vi "STED Control V7.vi"() -> ()   [LabVIEW 2014]
uses:
  Type Defs/Image Acquisition Parameters.ctl
  Laser Controls.ctl
  Detectors.ctl
  Type Defs/P541.ctl
  Type Defs/M227.ctl
  Type Defs/P612.ctl
  Type Defs/M686.ctl
  Type Defs/P841.ctl
  Type Defs/ASI.ctl
  Type Defs/N664_V2.ctl
  Type Defs/STED Graph Controls.ctl
  Type Defs/Display Controls.ctl
  FPGA-7842R-Reference.ctl
  Manual Controls V2.ctl
  Scan Parameters.ctl
  <vilib>/Utility/miscctls.llb/LVPositionTypeDef.ctl
  Controls/StageStates.ctl
  <vilib>/Utility/miscctls.llb/LVRectTypeDef.ctl
  <vilib>/Utility/cursorutil.llb/Set Cursor (Icon Pict).vi
panel:
  in  "Test":bool
  in  "Display Controls":T1
  in  "Graph Tools":T2
  in  "Shutters":T3
  in  "Upper Objective Z - N664":T4={"Up N664"=FALSE, "Down N664"=FALSE, "Step Size (um)"=0.001, "Position (mm)"=0.0} {"Step Size (um)" min=0.001}
  in  "Load Positions":bool
  in  "Cavity Translation Z - ASI":T5={"Up ASI"=FALSE, "Down ASI"=FALSE, "Step Size (um)"=0.001, "Z (um)"=0.001, "F (um)"=0.001, "Velocity"=0.001} caption="ASI" {"Velocity" min=0.001; "F (um)" min=0.001; "Z (um)" min=-1500.0 max=1500.0; "Step Size (um)" min=0.001}
  in  "Phase Comp Mirror - P841":T6={"Position (µm)"=0.0, "Step Size (µm)"=1.0, "Up P841"=FALSE, "Down P841"=FALSE}
  in  "Sample Stage XY - M686":T7 {"Y" format="%#_4g"; "X" format="%#_4g"}
  in  "Joystick Velocity":string(combo)
  in  "Radio Buttons":enum32{"Radio Selection 1", "Radio Selection 2"}(radio)
  in  "Bottom Objective XY - P612":T8 {"Y" format="%#_4g"; "X" format="%#_4g"}
  in  "Abort AllStage":bool
  in  "Stages":T9={"M227"=TRUE, "N664"=TRUE, "P612"=TRUE, "M686"=TRUE, "P841"=TRUE, "ASI"=TRUE}
  in  "Sample Z Coarse - M227":T10
  in  "Colormap":T11(ring)
  in  "Tab Control":T12(tab)
  in  "SLM":bool
  in  "DM":bool
  in  "Timing":bool
  in  "Sample Z - P541":T13={"Step Up"=FALSE, "Step Down"=FALSE, "Z Position"=0.0, "Step Size (um)"=1.0}
  out "Channel 6":sgl[][](graph)
  out "Channel 5":sgl[][](graph)
  out "Channel 4":sgl[][](graph)
  out "Channel 3":sgl[][](graph)
  out "Channel 2":sgl[][](graph)
  in  "Detectors":T14
  in  "Laser Controls":T15 {"STED Power (V)" scale=0.0..10.0}
  in  "Save File Path":path=path "C:/Users/ED STED/Desktop/temp.DBL"
  in  "Capture":bool
  out "Channel 1":sgl[][](graph)
  in  "Image Acquisition Parameters":T16={"Scan Type"=enum."Beam Scanning", "Scan Mode"=enum."XY", "Fast Axis Frequency (Hz)"=15780.0, "Image Format"=256, "Line Accumulations"=100, "Frames Per Capture"=1, "Frames Accumulations"=1, "Image Dimension (um)"=[15.0, 15.0], "Number of Z Steps"=1, "Z Steps Size (um)"=1.0, "Pixel Size (nm)"=[58.59375, 58.59375]} {"Z Steps Size (um)" min=0.0; "Number of Z Steps" min=1; "Frames Accumulations" min=1; "Frames Per Capture" min=1; "Line Accumulations" min=1; "Image Format" items=["64 x 64"=64, "128 x 128"=128, "256 x 256"=256, "512 x 512"=512, "1024 x 1024"=1024, "2048 x 2048"=2048]}
  in  "Live":bool
  in  "Exit":bool
  # "Sample Stage XY - M686 (0~25 mm)"
  # "XY"
  # "Z"
  # "Length"
  # "Height"
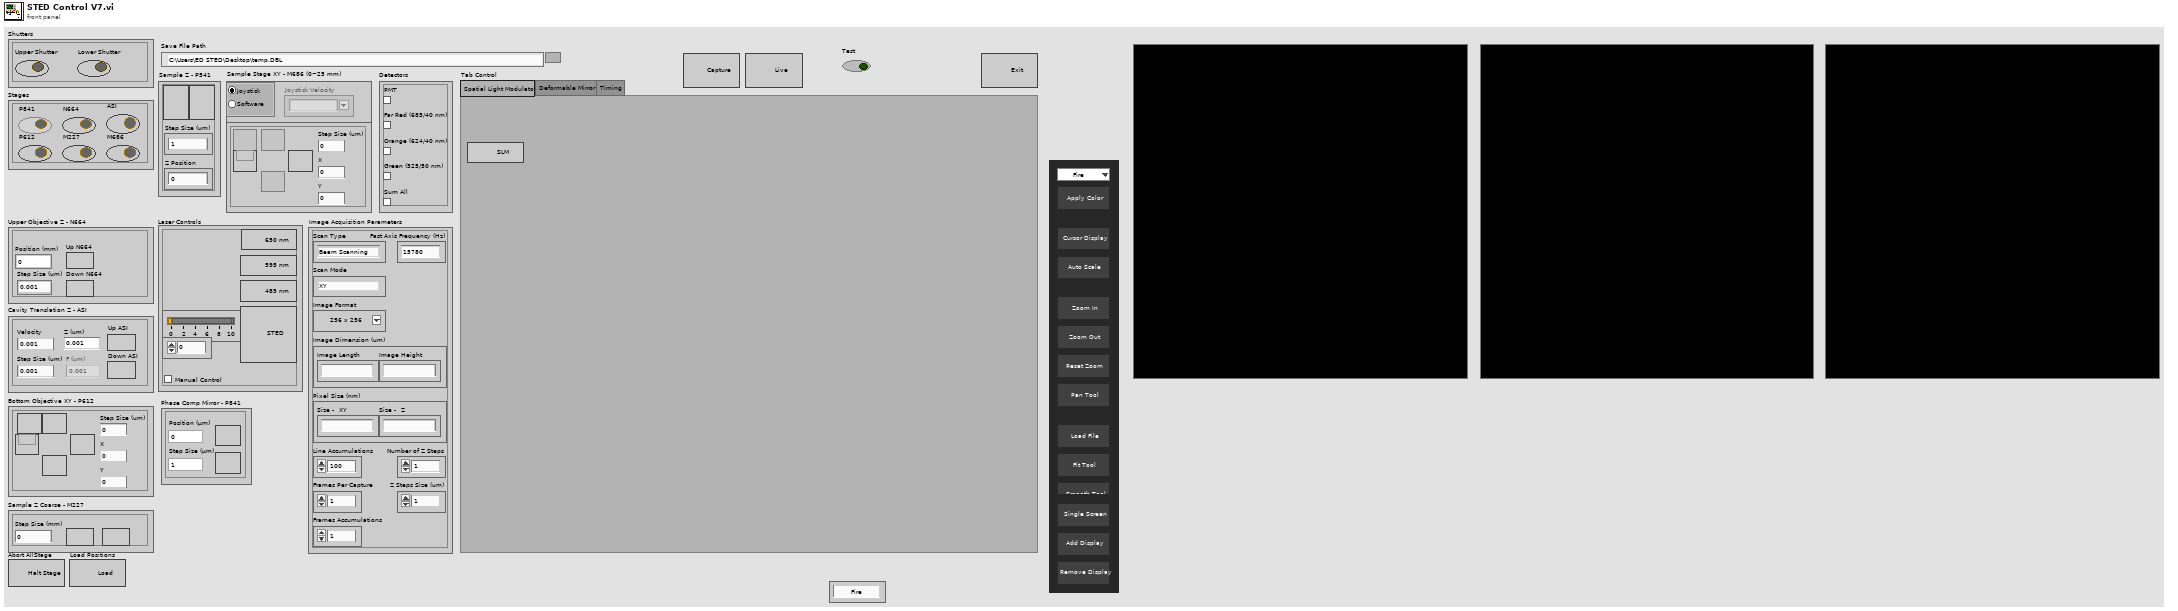
[diagram p1: front panel]
types:
  T1 = typedef "Display Controls.ctl" = cluster{"Remove Display":bool, "Add Display":bool, "Single Screen":bool}
  T2 = typedef "STED Graph Controls.ctl" = cluster{"Zoom Out":bool, "Zoom In":bool, "Reset Zoom":bool, "Pan Tool":bool, "Show Cursor":bool, "Load File":bool, "Fit Tool":bool, "Smooth Tool":bool, "Merge Tool":bool, "Auto Scale":bool, "Apply Color":bool, "Color Map":enum16{"Fire", "Gray", "Red", "Green", "Blue", "Cyan", "Magenta", "Yellow", "Red-White", "Green-White", "Blue-White", "Glow"}}
  T3 = cluster{"Upper Shutter":bool, "Lower Shutter":bool}
  T4 = typedef "N664_V2.ctl" = cluster{"Up N664":bool, "Down N664":bool, "Step Size (um)":dbl, "Position (mm)":dbl}
  T5 = typedef "ASI.ctl" = cluster{"Up ASI":bool, "Down ASI":bool, "Step Size (um)":dbl, "Z (um)":dbl, "F (um)":dbl, "Velocity":dbl}
  T6 = typedef "P841.ctl" = cluster{"Position (µm)":dbl, "Step Size (µm)":dbl, "Up P841":bool, "Down P841":bool}
  T7 = typedef "M686.ctl" = cluster{"Home Button":bool, "Up Button":bool, "Left Button":bool, "Down Button":bool, "Right Button":bool, "Step Size (um)":dbl, "X":dbl, "Y":dbl}
  T8 = typedef "P612.ctl" = cluster{"Home Button":bool, "Up Button":bool, "Left Button":bool, "Down Button":bool, "Right Button":bool, "Step Size (um)":dbl, "X":dbl, "Y":dbl}
  T9 = cluster{"M227":bool, "N664":bool, "P612":bool, "M686":bool, "P841":bool, "ASI":bool}
  T10 = typedef "M227.ctl" = cluster{"Up M227":bool, "Down M227":bool, "Step Size (mm)":dbl}
  T11 = enum16{"Fire", "Gray", "Red", "Green", "Blue", "Cyan", "Magenta", "Yellow", "Red-White", "Green-White", "Blue-White", "Glow"}
  T12 = enum32{"Spatial Light Modulator", "Deformable Mirror", "Timing"}
  T13 = typedef "P541.ctl" = cluster{"Step Up":bool, "Step Down":bool, "Z Position":dbl, "Step Size (um)":dbl}
  T14 = typedef "Detectors.ctl" = cluster{"PMT":bool, "Far Red (685/40 nm)":bool, "Orange (624/40 nm)":bool, "Green (525/50 nm)":bool, "Sum All":bool}
  T15 = typedef "Laser Controls.ctl" = cluster{"STED Power (V)":dbl, "STED":bool, "640 nm":bool, "590 nm":bool, "485 nm":bool, "Manual Control":bool}
  T16 = typedef "Image Acquisition Parameters.ctl" = cluster{"Scan Type":enum16{"Sample Scanning", "Beam Scanning"}, "Scan Mode":enum16{"XY", "XZ", "YZ", "XYZ"}, "Fast Axis Frequency (Hz)":dbl, "Image Format":u16, "Line Accumulations":u16, "Frames Per Capture":u16, "Frames Accumulations":u16, "Image Dimension (um)":dbl[], "Number of Z Steps":u8, "Z Steps Size (um)":dbl, "Pixel Size (nm)":dbl[]}
  T17 = typedef "Scan Parameters.ctl" = cluster{"Fast_Ax_Amp_V":dbl, "Fast_Ax_Off_V":dbl, "Slow_Ax_Amp_V":dbl, "Slow_Ax_Off_V ":dbl, "Slow_Ax_Max_V_VperS":dbl, "Slow_Ax1_Del25ns":i32, "Slow_Ax2_Del25ns":i32, "Stage_X_Off_V":dbl, "Stage_Y_Off_V":dbl, "Stage_Z_Off_V":dbl, "Galvo1_Off_V":dbl, "Galvo2_Off_V":dbl, "Last_Scan_Mode":enum16{"XY", "XZ", "YZ", "XYZ"}, "Current_Scan_Mode":enum16{"XY", "XZ", "YZ", "XYZ"}, "Fly_Back_Lines":u16, "Linear_Ramp_End":u32, "Z_Step_I16":i16, "Z_Start_I16":i16, "Laser_States _U32":u32, "590_Voltage_I16":i16, "775_AOM_Volt_I16":i16, "Blanking OFF":bool, "Unused_Axis_I16":i16}
  T18 = typedef "Manual Controls V2.ctl" = cluster{"Galvo 1 Position (I16)":i16, "Galvo 2 Position (I16)":i16, "X Axis Voltage (I16)":i16, "Y Axis Voltage (I16)":i16, "Z Axis Voltage (I16)":i16, "Res Mirror Amp (I16)":i16, "Res Mirror Mute":bool, "Upper Shutter":bool, "Lower Shutter":bool}
  T19 = typedef "FPGA-7842R-Reference.ctl" = enum16{"Stage Control", "Laser Control", "Unused Axis I16", "Exit", "Set Res Mirror", "Set Galvo", "Default", "Close FPGA", "Stop Waveforms", "Start Waveforms", "Shutter Control", "Initialize"}
  T20 = enum8{"Enabled", "Disabled", "Disabled and Grayed Out"}
  T21 = typedef "StageStates.ctl" = enum16{"POSITION", "MVR", "MOVE", "HALT", "ONTARGET", "ERROR", "EXIT", "HOME", "ZEROPOS", "NANOPOS", "QUIT", "ANALOG"}
  T22 = typedef "LVRectTypeDef.ctl" = cluster{"Left":i16, "Top":i16, "Right":i16, "Bottom":i16}
  T23 = enum32{"Invalid", "Standard", "Closed", "Hidden", "Minimized", "Maximized"}
  T24 = enum16{"open", "open or create", "create or replace", "create", "open (read-only)"}
  T25 = cluster{"Upper Shutter":bool, "Upper Shutter":bool}
  T26 = cluster{"Down_N664":bool, "Down_N664":bool, "Step Size (um)":dbl, "Numeric":dbl}
  T27 = cluster{bool, bool, bool, bool, bool, dbl, "Numeric":dbl, "Numeric":dbl}
  T28 = cluster{"Scan Type":bool, "Scan Mode":bool, "Fast Axis Frequency (Hz)":bool, "Image Format":bool, "Line Accumulations":bool, "Frames Per Capture":bool, "Frames Accumulations":bool, "Image Dimension (um)":bool[], "Number of Z Steps":bool, "Z Steps Size (um)":bool, "Pixel Size (nm)":bool[]}
  T29 = typedef "LVAllMonitorsDisplayTypeDef.ctl" = cluster{"Bounds":cluster{"Left":i16, "Top":i16, "Right":i16, "Bottom":i16}, "Depth":i16}[]
  T30 = cluster{"Bounds":cluster{"Left":i16, "Top":i16, "Right":i16, "Bottom":i16}, "Depth":i16}
  T31 = typedef "LVPositionTypeDef.ctl" = cluster{"Left":i32, "Top":i32}
  T32 = typedef "IMAQ Image.ctl" = refnum<image>
  T33 = typedef "Waveform Data.ctl" = cluster{"Waveform Scan Parameters":cluster{"Scanning Mode":u8, "Fast Axis WF Length (Elements)":i32, "Fast Axis Sample Period (Ticks)":u32, "Slow Axis 1 WF Length (Elements)":i32, "Slow Axis 1 Sample Period (Ticks)":u32, "Slow Axis 1 Delay (25 ns) Steps":i32, "Slow Axis 2 WFLength (Elements)":i32, "Slow Axis 2 Sample Period (Ticks)":u32, "Slow Axis 2 Delay (25 ns) Steps":i32}, "Fast Axis Waveform":dbl[], "Slow Axis 1 Waveform":dbl[], "Slow Axis 2 Waveform":dbl[]}
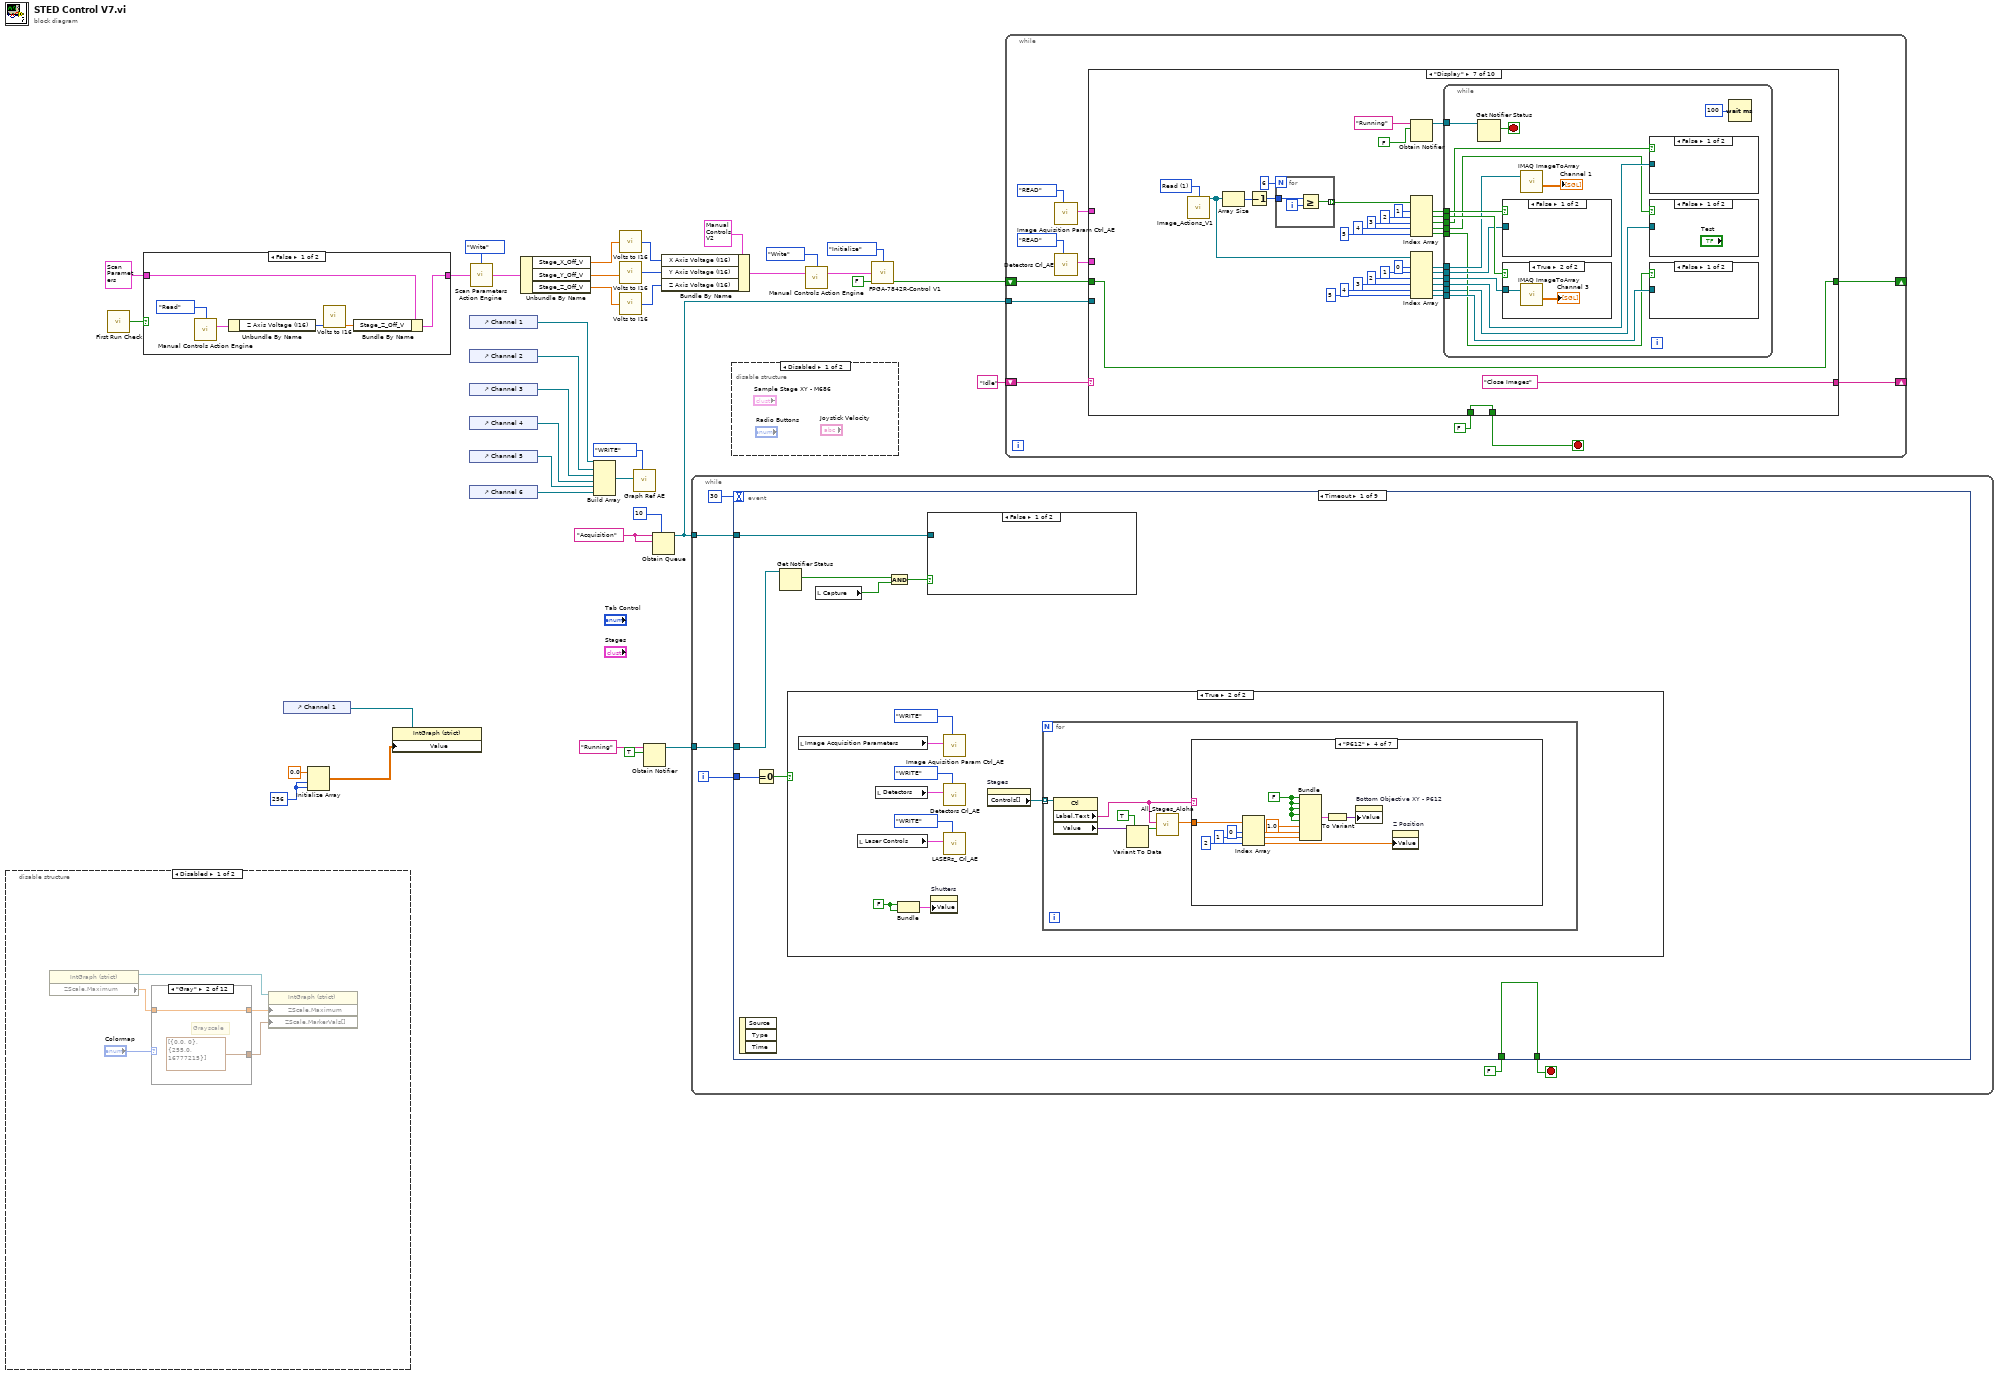
[diagram p0: block diagram]
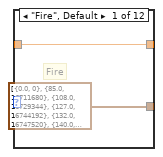
[diagram p2: hidden frame]
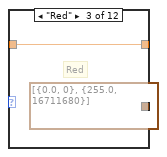
[diagram p3: hidden frame]
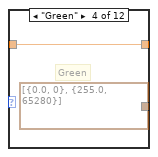
[diagram p4: hidden frame]
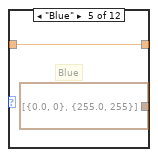
[diagram p5: hidden frame]
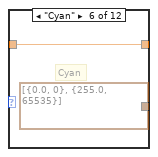
[diagram p6: hidden frame]
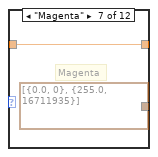
[diagram p7: hidden frame]
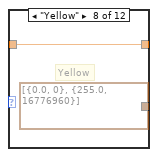
[diagram p8: hidden frame]
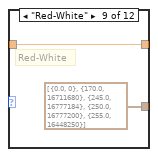
[diagram p9: hidden frame]
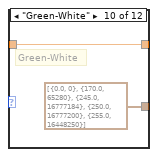
[diagram p10: hidden frame]
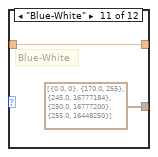
[diagram p11: hidden frame]
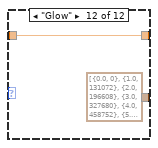
[diagram p12: hidden frame]
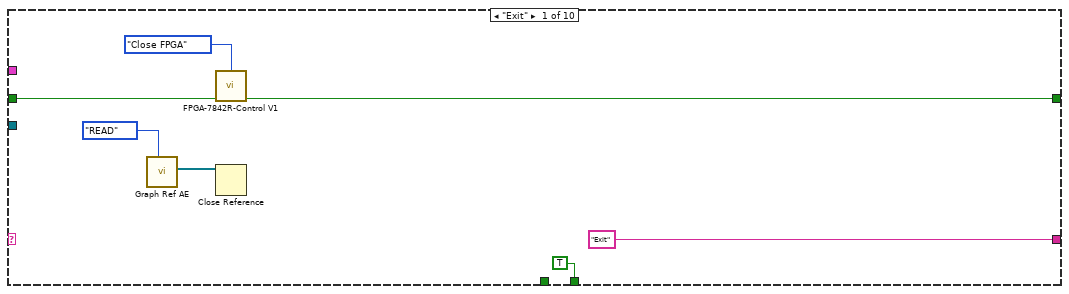
[diagram p16: hidden frame]
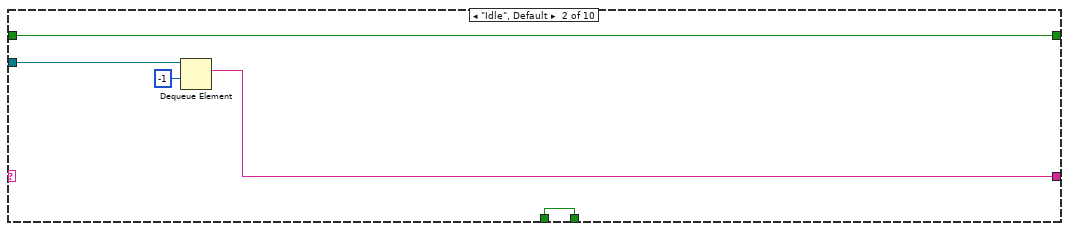
[diagram p17: hidden frame]
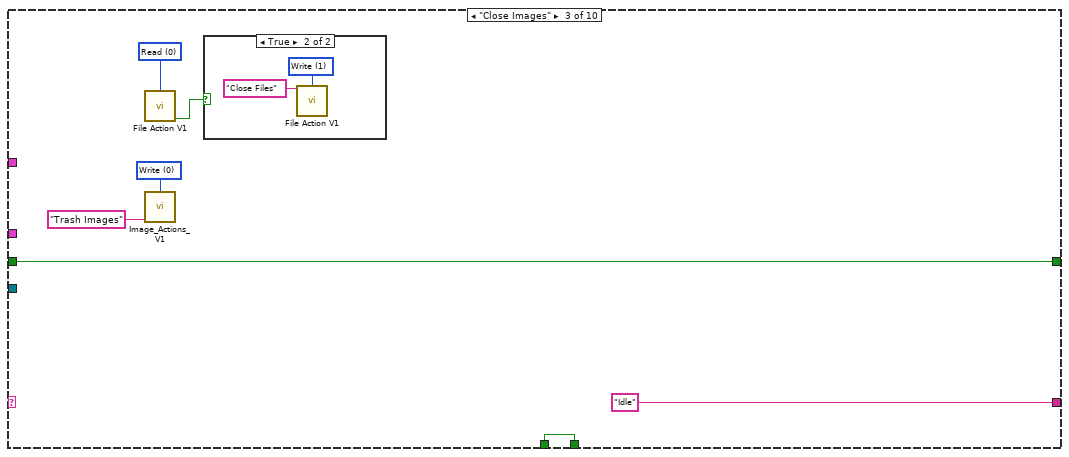
[diagram p18: hidden frame]
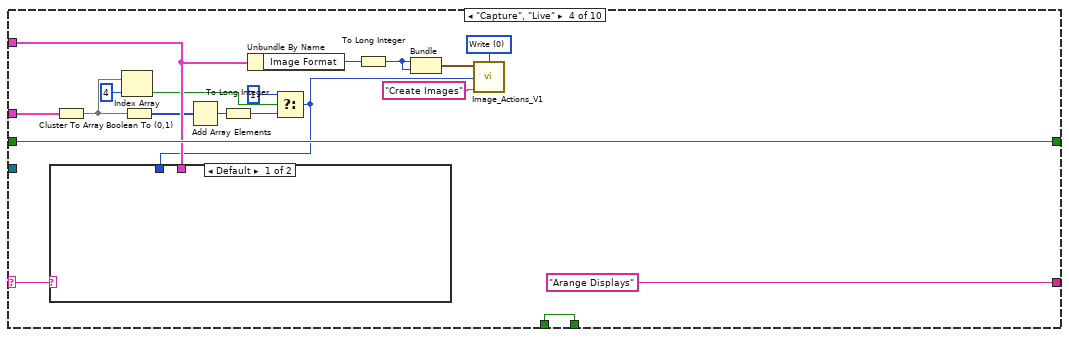
[diagram p20: hidden frame]
diagram:
  w3 = 256 ("dimension size")
  w14 = "Acquisition" ("name (unnamed)")
  n1 = disable-structure shown="Disabled" {
    frame Disabled {
      n2 = property class="IntGraph (strict)"() -> (reference out=w40:refnum<vi>, "ZScale.Maximum"=w39:dbl)  [unwired: 2 in, 1 out]
      n3 = case shown="\"Gray\"" "Colormap" {
        tunnel: [cluster{dbl, u32}[] [{0.0, 0}, {85.0, 16711680}, {108.0, 16729344}, {127.0, 16744192}, {132.0, 16747520}, {140.0, 16753920}, {157.0, 16766720}, {170.0, 16776960}, {245.0, 16777184}, {250.0, 16777200}, {255.0, 16777215}] ("Z Scale.Marker Values[]") cluster{dbl, u32}[] [{0.0, 0}, {255.0, 16777215}] ("Z Scale.Marker Values[]") cluster{dbl, u32}[] [{0.0, 0}, {255.0, 16711680}] ("Z Scale.Marker Values[]") cluster{dbl, u32}[] [{0.0, 0}, {255.0, 65280}] ("Z Scale.Marker Values[]") cluster{dbl, u32}[] [{0.0, 0}, {255.0, 255}] ("Z Scale.Marker Values[]") cluster{dbl, u32}[] [{0.0, 0}, {255.0, 65535}] ("Z Scale.Marker Values[]") cluster{dbl, u32}[] [{0.0, 0}, {255.0, 16711935}] ("Z Scale.Marker Values[]") cluster{dbl, u32}[] [{0.0, 0}, {255.0, 16776960}] ("Z Scale.Marker Values[]") cluster{dbl, u32}[] [{0.0, 0}, {170.0, 16711680}, {245.0, 16777184}, {250.0, 16777200}, {255.0, 16448250}] ("Z Scale.Marker Values[]") cluster{dbl, u32}[] [{0.0, 0}, {170.0, 65280}, {245.0, 16777184}, {250.0, 16777200}, {255.0, 16448250}] ("Z Scale.Marker Values[]") cluster{dbl, u32}[] [{0.0, 0}, {170.0, 255}, {245.0, 16777184}, {250.0, 16777200}, {255.0, 16448250}] ("Z Scale.Marker Values[]") cluster{dbl, u32}[] [{0.0, 0}, {1.0, 131072}, {2.0, 196608}, {3.0, 327680}, {4.0, 458752}, {5.0, 589824}, {6.0, 720896}, {7.0, 851971}, {8.0, 983043}, {9.0, 1114115}, {10.0, 1245187}, {11.0, 1376259}, {12.0, 1507331}, {13.0, 1638403}, {14.0, 1769475}, {15.0, 1769479}, {16.0, 2031623}, {17.0, 2162695}, {18.0, 2293767}, {19.0, 2424839}, {20.0, 2555911}, {21.0, 2686983}, {22.0, 2818055}, {23.0, 2949127}, {24.0, 3080203}, {25.0, 3211275}, {26.0, 3342347}, {27.0, 3473419}, {28.0, 3604491}, {29.0, 3735563}, {30.0, 3866635}, {31.0, 3867403}, {32.0, 4129547}, {33.0, 4260619}, {34.0, 4391691}, {35.0, 4522763}, {36.0, 4653839}, {37.0, 4784911}, {38.0, 4915983}, {39.0, 5178127}, {40.0, 5309199}, {41.0, 5440271}, {42.0, 5571343}, {43.0, 5702415}, {44.0, 5703439}, {45.0, 5965583}, {46.0, 6096655}, {47.0, 6227727}, {48.0, 6358799}, {49.0, 6489871}, {50.0, 6620943}, {51.0, 6752015}, {52.0, 6883087}, {53.0, 7015183}, {54.0, 7146255}, {55.0, 7277327}, {56.0, 7408399}, {57.0, 7539471}, {58.0, 7670543}, {59.0, 7801615}, {60.0, 8063759}, {61.0, 8194831}, {62.0, 8326927}, {63.0, 8457999}, {64.0, 8589075}, {65.0, 8720147}, {66.0, 8851219}, {67.0, 8982291}, {68.0, 9113363}, {69.0, 9114387}, {70.0, 9376531}, {71.0, 9507603}, {72.0, 9638675}, {73.0, 9769747}, {74.0, 9901843}, {75.0, 10032915}, {76.0, 10163987}, {77.0, 10229523}, {78.0, 10295059}, {79.0, 10427155}, {80.0, 10558227}, {81.0, 10689299}, {82.0, 10820371}, {83.0, 10886931}, {84.0, 10952467}, {85.0, 11083539}, {86.0, 11214611}, {87.0, 11215635}, {88.0, 11477779}, {89.0, 11543315}, {90.0, 11608851}, {91.0, 11740947}, {92.0, 11806483}, {93.0, 11872019}, {94.0, 12004115}, {95.0, 12135187}, {96.0, 12266259}, {97.0, 12267283}, {98.0, 12398355}, {99.0, 12529427}, {100.0, 12530451}, {101.0, 12595987}, {102.0, 12530451}, {103.0, 12793619}, {104.0, 12794131}, {105.0, 12794643}, {106.0, 13056787}, {107.0, 13057299}, {108.0, 13057811}, {109.0, 13188883}, {110.0, 13320979}, {111.0, 13386515}, {112.0, 13452563}, {113.0, 13584147}, {114.0, 13584659}, {115.0, 13585171}, {116.0, 13585683}, {117.0, 13717267}, {118.0, 13848339}, {119.0, 13849363}, {120.0, 13849875}, {121.0, 13850387}, {122.0, 13981459}, {123.0, 14113555}, {124.0, 14114067}, {125.0, 14114579}, {126.0, 14115091}, {127.0, 14246675}, {128.0, 14377747}, {129.0, 14378771}, {130.0, 14379283}, {131.0, 14379539}, {132.0, 14379795}, {133.0, 14380819}, {134.0, 14511891}, {135.0, 14643987}, {136.0, 14644503}, {137.0, 14645015}, {138.0, 14645527}, {139.0, 14646039}, {140.0, 14646551}, {141.0, 14778135}, {142.0, 14909207}, {143.0, 14910231}, {144.0, 14910747}, {145.0, 14911259}, {146.0, 14911771}, {147.0, 14912283}, {148.0, 14912797}, {149.0, 15044383}, {150.0, 15175455}, {151.0, 15175967}, {152.0, 15176479}, {153.0, 15176991}, {154.0, 15177507}, {155.0, 15178019}, {156.0, 15178531}, {157.0, 15310115}, {158.0, 15441701}, {159.0, 15441959}, {160.0, 15442215}, {161.0, 15442727}, {162.0, 15443243}, {163.0, 15443755}, {164.0, 15444269}, {165.0, 15444783}, {166.0, 15444783}, {167.0, 15576367}, {168.0, 15707953}, {169.0, 15708467}, {170.0, 15708979}, {171.0, 15708981}, {172.0, 15708983}, {173.0, 15710011}, {174.0, 15710523}, {175.0, 15711037}, {176.0, 15711039}, {177.0, 15711553}, {178.0, 15843139}, {179.0, 15974213}, {180.0, 15974215}, {181.0, 15974217}, {182.0, 15974219}, {183.0, 15975755}, {184.0, 15976271}, {185.0, 15976785}, {186.0, 15977299}, {187.0, 15977301}, {188.0, 15977815}, {189.0, 15978327}, {190.0, 15978331}, {191.0, 16109917}, {192.0, 16241503}, {193.0, 16241505}, {194.0, 16242019}, {195.0, 16242535}, {196.0, 16242537}, {197.0, 16242539}, {198.0, 16243563}, {199.0, 16243567}, {200.0, 16244081}, {201.0, 16244595}, {202.0, 16244599}, {203.0, 16244601}, {204.0, 16244603}, {205.0, 16245627}, {206.0, 16245631}, {207.0, 16245633}, {208.0, 16246147}, {209.0, 16246663}, {210.0, 16377735}, {211.0, 16508811}, {212.0, 16508815}, {213.0, 16509839}, {214.0, 16509843}, {215.0, 16509845}, {216.0, 16509847}, {217.0, 16510361}, {218.0, 16510875}, {219.0, 16510879}, {220.0, 16510881}, {221.0, 16510883}, {222.0, 16511399}, {223.0, 16511911}, {224.0, 16511915}, {225.0, 16511917}, {226.0, 16511919}, {227.0, 16511923}, {228.0, 16512437}, {229.0, 16512951}, {230.0, 16512955}, {231.0, 16512957}, {232.0, 16512959}, {233.0, 16512961}, {234.0, 16512963}, {235.0, 16512967}, {236.0, 16513481}, {237.0, 16513995}, {238.0, 16513999}, {239.0, 16514001}, {240.0, 16514003}, {241.0, 16514005}, {242.0, 16514007}, {243.0, 16514011}, {244.0, 16514013}, {245.0, 16514015}, {246.0, 16514019}, {247.0, 16514021}, {248.0, 16514023}, {249.0, 16514027}, {250.0, 16514029}, {251.0, 16514031}, {252.0, 16514035}, {253.0, 16514037}, {254.0, 16514039}, {255.0, 16514043}] ("Z Scale.Marker Values[]")] -> w42
        tunnel: [w43 w45 w47 w49 w51 w53 w55 w57 w59 w61 w63 w65] -> w41
        tunnel: w39 -> [w43 w45 w47 w49 w51 w53 w55 w57 w59 w61 w63 w65]
        frame "Fire", Default {
          # "Fire"
        }
        frame "Gray" {
          # "Grayscale"
        }
        frame "Red" {
          # "Red"
        }
        frame "Green" {
          # "Green"
        }
        frame "Blue" {
          # "Blue"
        }
        frame "Cyan" {
          # "Cyan"
        }
        frame "Magenta" {
          # "Magenta"
        }
        frame "Yellow" {
          # "Yellow"
        }
        frame "Red-White" {
          # "Red-White"
        }
        frame "Green-White" {
          # "Green-White"
        }
        frame "Blue-White" {
          # "Blue-White"
        }
        frame "Glow" {
        }
      }
      n4 = property class="IntGraph (strict)"(reference=w40, "ZScale.Maximum"=w41, "ZScale.MarkerVals[]"=w42) -> ()  [unwired: 1 in, 2 out]
    }
    frame Enabled {
    }
  }
  n5 = call "First Run Check.vi"() -> ("First Run?"=w7:bool)  [unwired: 15 in]
  n6 = case shown="False" w7 {
    tunnel: T17 {"Fast_Ax_Amp_V"=0.0, "Fast_Ax_Off_V"=0.0, "Slow_Ax_Amp_V"=0.0, "Slow_Ax_Off_V "=0.0, "Slow_Ax_Max_V_VperS"=0.0, "Slow_Ax1_Del25ns"=0, "Slow_Ax2_Del25ns"=0, "Stage_X_Off_V"=5.0, "Stage_Y_Off_V"=5.0, "Stage_Z_Off_V"=5.0, "Galvo1_Off_V"=0.0, "Galvo2_Off_V"=0.0, "Last_Scan_Mode"=enum."XY", "Current_Scan_Mode"=enum."XY", "Fly_Back_Lines"=0, "Linear_Ramp_End"=0, "Z_Step_I16"=0, "Z_Start_I16"=0, "Laser_States _U32"=0, "590_Voltage_I16"=0, "775_AOM_Volt_I16"=0, "Blanking OFF"=FALSE, "Unused_Axis_I16"=16384} ("Scan Parameters IN") -> [w72 w73]
    tunnel: [w67 w73] -> w5
    frame False {
      n7 = call "Manual Controls Action Engine.vi"("Action"=enum16{"Read", "Write"}."Read") -> ("Manual Controls Out"=w70:T18)  [unwired: 14 in]
      n8 = Unbundle By Name(w70) -> ("Z Axis Voltage (I16)"=w71:i16)
      n9 = call "Volts to I16.vi"("Volatge (I16)"=w71) -> ("Voltage (V)"=w68:dbl)  [unwired: 13 in, 1 out]
      n10 = Bundle By Name(cluster=w72, "Stage_Z_Off_V"=w68) -> (w67:T17)
    }
    frame True {
    }
  }
  n11 = control-ref of="Channel 1"() -> (w4:refnum<vi>)
  n12 = Initialize Array(sgl 0.0 ("element"), w3, w3) -> (w1:sgl[][])
  n13 = property class="IntGraph (strict)"(reference=w4, "Value"=w1) -> ()  [unwired: 1 in, 2 out]
  n14 = control-ref of="Channel 1"() -> (w8:refnum<vi>)
  n15 = control-ref of="Channel 2"() -> (w34:refnum<vi>)
  n16 = control-ref of="Channel 3"() -> (w19:refnum<vi>)
  n17 = control-ref of="Channel 4"() -> (w33:refnum<vi>)
  n18 = control-ref of="Channel 5"() -> (w32:refnum<vi>)
  n19 = control-ref of="Channel 6"() -> (w31:refnum<vi>)
  n20 = call "Scan Parameters Action Engine.vi"("Action"=enum16{"Read", "Write"}."Write", "Scan Parameters IN"=w5) -> ("Scan Parameters OUT"=w26:T17)  [unwired: 13 in]
  n21 = Unbundle By Name(w26) -> ("Stage_X_Off_V"=w22:dbl, "Stage_Y_Off_V"=w21:dbl, "Stage_Z_Off_V"=w20:dbl)
  n22 = Build Array(w8, w34, w19, w33, w32, w31) -> (w17:refnum<vi>[])
  n23 = call "Volts to I16.vi"("Voltage (V)"=w22) -> ("I16"=w23:i16)  [unwired: 13 in, 1 out]
  n24 = call "Volts to I16.vi"("Voltage (V)"=w21) -> ("I16"=w24:i16)  [unwired: 13 in, 1 out]
  n25 = call "Volts to I16.vi"("Voltage (V)"=w20) -> ("I16"=w25:i16)  [unwired: 13 in, 1 out]
  n26 = call "Graph Ref AE.vi"("Action"=enum16{"READ", "WRITE"}."WRITE", "Graph Ref In"=w17) -> ()  [unwired: 9 in, 1 out]
  n27 = Obtain Notifier(name (unnamed)="Running", notification data type=TRUE) -> (notifier out=w10:refnum<notifier>)  [unwired: 2 in, 2 out]
  n28 = Obtain Queue(max queue size (-1, unlimited)=10, name (unnamed)=w14, element data type=w14) -> (queue out=w16:refnum<queue>)  [unwired: 2 in, 2 out]
  n29 = Bundle By Name(cluster=T18 {"Galvo 1 Position (I16)"=-280, "Galvo 2 Position (I16)"=0, "X Axis Voltage (I16)"=16384, "Y Axis Voltage (I16)"=16384, "Z Axis Voltage (I16)"=16384, "Res Mirror Amp (I16)"=0, "Res Mirror Mute"=FALSE, "Upper Shutter"=FALSE, "Lower Shutter"=FALSE} ("Manual Controls"), "X Axis Voltage (I16)"=w23, "Y Axis Voltage (I16)"=w24, "Z Axis Voltage (I16)"=w25) -> (w27:T18)
  n30 = while {
    tunnel: w16 -> [w77]
    tunnel: w10 -> [w74]
    i -> [w75]
    stop <- w79 stop-if-true
    n31 = event shown="[0] Timeout" {
      selector: _ -> [_ _ _ _ _ _ _ _ _]
      dyn-events: _ -> [_ _ _ _ _ _ _ _ _]
      timeout: 30 -> [_ _ _ _ _ _ _ _ _]
      tunnel: [w87 w187 w200 w323 w552 w603 _ w784 w885] -> w79
      tunnel: FALSE -> [w87 w187 w200 w323 w552 w603 _ w784 _]
      tunnel: w77 -> [w84 w186 _ _ _ _ _ _ w884]
      tunnel: w75 -> [w82 _ _ _ _ _ _ _ _]
      tunnel: w74 -> [w80 w179 _ _ _ _ _ _ w878]
      event Timeout {
        n32 = event-data() -> ()  [unwired: 1 in, 3 out]
        n33 = Equal To 0?(x=w82) -> (x = 0?=w81:bool)
        n34 = Get Notifier Status(notifier=w80) -> (current notification=w86:bool)  [unwired: 1 in, 4 out]
        n35 = case shown="True" w81 {
          frame False {
            w92 = enum16{"WRITE", "READ"}."READ" ("Enum")
            n36 = call "Image Aquisition Param Ctrl_AE.vi"("Action"=enum16{"READ", "WRITE"}."READ") -> ("Image Acquisition Parameters Out"=w108:T16)  [unwired: 10 in]
            n37 = call "Detectors Crl_AE.vi"("Action"=enum16{"READ", "WRITE"}."READ") -> ("Detectors Parameters Out"=w109:T14)  [unwired: 10 in]
            n38 = call "LASERs_ Crl_AE.vi"("Action"=enum16{"READ", "WRITE"}."READ") -> ("Detectors Parameters Out"=w110:T15)  [unwired: 10 in]
            n39 = local write "Image Acquisition Parameters"(w108) -> ()
            n40 = local write "Detectors"(w109) -> ()
            n41 = local write "Laser Controls"(w110) -> ()
            n42 = call "Stage_position_ae.vi"("StageID"="P612", "Enum"=w92) -> ("Position Out"=w103:dbl[])  [unwired: 8 in, 1 out]
            n43 = call "Stage_position_ae.vi"("StageID"="P841", "Enum"=w92) -> ("Position Out"=w96:dbl[])  [unwired: 8 in, 1 out]
            n44 = call "Stage_position_ae.vi"("StageID"="N664", "Enum"=w92) -> ("Position Out"=w89:dbl[])  [unwired: 8 in, 1 out]
            n45 = Index Array(array=w89, index=0) -> (element=w88:dbl)
            n46 = Index Array(array=w96, index=0) -> (element=w93:dbl)
            n47 = Index Array(array=w103, index #1=0 ("index"), index #2=1 ("index"), index #3=2 ("index")) -> (element #1=w102:dbl, element #2=w99:dbl, element #3=w97:dbl)
            n48 = property on="Position (µm)" class="DigNum (strict)"("Value"=w93) -> ()  [unwired: 2 in, 2 out]
            n49 = property on="Position (mm)" class="DigNum (strict)"("Value"=w88) -> ()  [unwired: 2 in, 2 out]
            n50 = property on="X" class="DigNum (strict)"("Value"=w102) -> ()  [unwired: 2 in, 2 out]
            n51 = property on="Y" class="DigNum (strict)"("Value"=w99) -> ()  [unwired: 2 in, 2 out]
            n52 = property on="Z Position" class="DigNum (strict)"("Value"=w97) -> ()  [unwired: 2 in, 2 out]
          }
          frame True {
            w111 = FALSE ("Upper Shutter")
            n53 = local read "Image Acquisition Parameters"() -> (w118:T16)
            n54 = local read "Laser Controls"() -> (w116:T15)
            n55 = local read "Detectors"() -> (w115:T14)
            n56 = Bundle("Upper Shutter"=w111, "Upper Shutter"=w111) -> (w112:T25)  [unwired: 1 in]
            n57 = property on="Shutters" class="Clust (strict)"("Value"=w112) -> ()  [unwired: 2 in, 2 out]
            n58 = call "Image Aquisition Param Ctrl_AE.vi"("Action"=enum16{"READ", "WRITE"}."WRITE", "Image Acquisition Parameters In"=w118) -> ()  [unwired: 9 in, 1 out]
            n59 = call "Detectors Crl_AE.vi"("Action"=enum16{"READ", "WRITE"}."WRITE", "Detectors Parameters In"=w115) -> ()  [unwired: 9 in, 1 out]
            n60 = call "LASERs_ Crl_AE.vi"("Action"=enum16{"READ", "WRITE"}."WRITE", "Detectors Parameters In"=w116) -> ()  [unwired: 9 in, 1 out]
            n61 = property on="Stages" class="Clust (strict)"() -> ("Controls[]"=w113:refnum<vi>[])  [unwired: 2 in, 2 out]
            n62 = for {
              tunnel: w113 -> [w123] mode=indexing
              n63 = property class="Ctl"(reference=w123) -> ("Label.Text"=w121:string, "Value"=w125:variant)  [unwired: 1 in, 2 out]
              n64 = Variant To Data(type=TRUE, Variant=w125) -> (data=w122:bool)  [unwired: 1 in, 1 out]
              n65 = call "All_Stages_Aloha.vi"("Aloha"=w122, "Stage ID"=w121) -> ("Position Out"=w120:dbl[])  [unwired: 9 in]
              n66 = case shown="\"P612\"" w121 {
                tunnel: w120 -> [_ _ w132 w139 w149 w160 w170]
                frame "0", Default {
                }
                frame "M227" {
                  w129 = FALSE
                  n67 = Bundle(w129, w129, 0.0) -> (w127:cluster{bool, bool, dbl})  [unwired: 1 in]
                  n68 = To Variant(anything=w127) -> (Variant=w126:variant)
                  n69 = property on="Sample Z Coarse - M227" class="Clust"("Value"=w126) -> ()  [unwired: 2 in, 2 out]
                }
                frame "N664" {
                  w135 = FALSE ("Down_N664")
                  n70 = Index Array(array=w132, index=0) -> (element=w133:dbl)
                  n71 = Bundle("Down_N664"=w135, "Down_N664"=w135, "Step Size (um)"=1.0, "Numeric"=w133) -> (w131:T26)  [unwired: 1 in]
                  n72 = To Variant(anything=w131) -> (Variant=w130:variant)
                  n73 = property on="Upper Objective Z - N664" class="Clust"("Value"=w130) -> ()  [unwired: 2 in, 2 out]
                }
                frame "P612" {
                  w147 = FALSE
                  n74 = Index Array(array=w139, index #1=0, index #2=1, index #3=2 ("index")) -> (element #1=w144:dbl, element #2=w142:dbl, element #3=w137:dbl)
                  n75 = Bundle(w147, w147, w147, w147, w147, 1.0, "Numeric"=w144, "Numeric"=w142) -> (w143:T27)  [unwired: 1 in]
                  n76 = To Variant(anything=w143) -> (Variant=w138:variant)
                  n77 = property on="Bottom Objective XY - P612" class="Clust"("Value"=w138) -> ()  [unwired: 2 in, 2 out]
                  n78 = property on="Z Position" class="DigNum (strict)"("Value"=w137) -> ()  [unwired: 2 in, 2 out]
                }
                frame "M686" {
                  w158 = FALSE
                  n79 = Index Array(array=w149, index #1=0, index #2=1) -> (element #1=w155:dbl, element #2=w150:dbl)
                  n80 = Bundle(w158, w158, w158, w158, w158, 10.0, "Numeric"=w155, "Numeric"=w150) -> (w154:T27)  [unwired: 1 in]
                  n81 = To Variant(anything=w154) -> (Variant=w148:variant)
                  n82 = property on="Joystick Velocity" class="CmbBox"("DisabledEnum"=T20."Disabled and Grayed Out" ("Disabled")) -> ()  [unwired: 2 in, 2 out]
                  n83 = property on="Radio Buttons" class="RadioBtnsControl (strict)"("Value"=enum32{"Radio Selection 1", "Radio Selection 2"}."Radio Selection 2" ("Radio Buttons")) -> ()  [unwired: 2 in, 2 out]
                  n84 = property on="Sample Stage XY - M686" class="Clust"("Value"=w148) -> ()  [unwired: 2 in, 2 out]
                }
                frame "P841" {
                  n85 = Index Array(array=w160, index=0) -> (element=w159:dbl)
                  n86 = property on="Position (µm)" class="DigNum (strict)"("Value"=w159) -> ()  [unwired: 2 in, 2 out]
                }
                frame "ASI" {
                  w166 = FALSE
                  n87 = Add Array Elements(numeric array=w170) -> (sum=w172:dbl)
                  n88 = Index Array(array=w170, index #1=0 ("index"), index #2=1 ("index")) -> (element #1=w165:dbl, element #2=w164:dbl)
                  n89 = Divide(x=w172, y=2000.0) -> ()  [unwired: 1 out]
                  n90 = Bundle By Name(cluster=T5 {"Up ASI"=FALSE, "Down ASI"=FALSE, "Step Size (um)"=0.001, "Z (um)"=0.001, "F (um)"=0.001, "Velocity"=0.001} ("Cavity Translation Z - ASI"), "Up ASI"=w166, "Down ASI"=w166, "Step Size (um)"=1.0, "Z (um)"=w165, "F (um)"=w164, "Velocity"=0.1) -> (w162:T5)
                  n91 = To Variant(anything=w162) -> (Variant=w163:variant)
                  n92 = property on="Cavity Translation Z - ASI" class="Clust"("Value"=w163) -> ()  [unwired: 2 in, 2 out]
                }
              }
            }
          }
        }
        n93 = local read "Capture"() -> (w85:bool)
        n94 = And(x=w86, y=w85) -> (x .and. y?=w83:bool)
        n95 = case shown="False" w83 {
          tunnel: w84 -> [_ w177]
          frame False {
          }
          frame True {
            n96 = local write "Capture"(FALSE ("Capture")) -> ()
            n97 = Enqueue Element(queue=w177, element="Stop Acquisition" ("f")) -> ()  [unwired: 2 in, 3 out]
            n98 = property on="Live" class="Bool (strict)"("DisabledEnum"=T20."Enabled" ("Disabled")) -> ()  [unwired: 2 in, 2 out]
          }
        }
      }
      event "Live", "Capture": Value Change {
        n99 = event-data() -> ("CtlRef"=w185:refnum<vi>, "NewVal"=w180:bool)  [unwired: 1 in]
        n100 = Not(x=w180) -> (.not. x?=w183:bool)
        n101 = property class="Bool (strict)"(reference=w185) -> ("Label.Text"=w181:string)  [unwired: 1 in, 2 out]
        n102 = Send Notification(notification=w183, notifier=w179) -> ()  [unwired: 1 in, 2 out]
        n103 = case shown="\"Capture\"" w181 {
          tunnel: w180 -> [_ w189 w193]
          frame "False", Default {
          }
          frame "Live" {
            n104 = case shown="True" w189 {
              tunnel: [T20."Enabled" ("Disabled") T20."Disabled and Grayed Out" ("Disabled")] -> w188
              frame False {
              }
              frame True {
              }
            }
            n105 = property on="Capture" class="Bool (strict)"("DisabledEnum"=w188) -> ()  [unwired: 2 in, 2 out]
            n106 = property on="Exit" class="Bool"("DisabledEnum"=w188) -> ()  [unwired: 2 in, 2 out]
          }
          frame "Capture" {
            n107 = case shown="True" w193 {
              tunnel: [T20."Enabled" ("Disabled") T20."Disabled and Grayed Out" ("Disabled")] -> w192
              frame False {
              }
              frame True {
              }
            }
            n108 = property on="Live" class="Bool (strict)"("DisabledEnum"=w192) -> ()  [unwired: 2 in, 2 out]
            n109 = property on="Exit" class="Bool"("DisabledEnum"=w192) -> ()  [unwired: 2 in, 2 out]
          }
        }
        n110 = Select(t=w181, s=w180, f="Stop Acquisition") -> (s? t:f=w182:string)
        n111 = Enqueue Element(queue=w186, element=w182) -> ()  [unwired: 2 in, 3 out]
      }
      event "Shutters": Value Change {
        n112 = event-data() -> ("CtlRef"=w199:refnum<vi>, "NewVal"=w198:variant, "OldVal"=w197:variant)  [unwired: 1 in]
        n113 = property class="Clust"(reference=w199) -> ("Label.Text"=w196:string)  [unwired: 1 in, 2 out]
        n114 = case shown="\"Shutters\"" w196 {
          tunnel: w198 -> [_ w205 _ _ _]
          tunnel: w197 -> [_ w203 _ _ _]
          frame Default {
          }
          frame "Image Acquisition Parameters" {
            n115 = Variant To Data(type="Image Acquisition Parameters", Variant=w205) -> (data=w202:T16)  [unwired: 1 in, 1 out]
            n116 = Variant To Data(type=w202, Variant=w203) -> (data=w201:T16)  [unwired: 1 in, 1 out]
            n117 = Not Equal?(x=w202, y=w201) -> (x != y?=w227:T28)
            n118 = Unbundle By Name(w227) -> ("Image Dimension (um)"=w212:bool[], "Image Format"=w210:bool, "Pixel Size (nm)"=w211:bool[])
            n119 = Or Array Elements(Boolean array=w212) -> (logical OR=w216:bool)
            n120 = Or Array Elements(Boolean array=w211) -> (logical OR=w215:bool)
            n121 = Build Array(w216, w210, w215) -> (w214:bool[])
            n122 = Boolean Array To Number(Boolean array=w214) -> (number=w213:u32)
            n123 = case shown="0, Default" w213 {
              tunnel: w212 -> [_ w251 _]
              tunnel: w202 -> [w239 w244 w259]
              tunnel: [w239 w242 w257] -> w209
              tunnel: w211 -> [_ _ w256]
              tunnel: [w238 w241 w255] -> w208
              tunnel: [w237 w240 w254] -> w206
              frame 0, Default {
                n124 = Unbundle By Name(w239) -> ("Image Dimension (um)"=w238:dbl[], "Scan Mode"=w237:enum16{"XY", "XZ", "YZ", "XYZ"})
              }
              frame 1, 2 {
                # "Image Dimension or Format Change"
                n125 = Unbundle By Name(w244) -> ("Image Dimension (um)"=w250:dbl[], "Image Format"=w248:u16, "Scan Mode"=w240:enum16{"XY", "XZ", "YZ", "XYZ"})
                n126 = for {
                  tunnel: w251 -> [w253] mode=indexing
                  tunnel: w250 -> [w252] mode=indexing
                  tunnel: [w252] -> w249
                  stop <- w253 stop-if-true
                }
                n127 = To Double Precision Float(number=w248) -> (double precision float=w247:dbl)
                n128 = Build Array(w249, w249) -> (w241:dbl[])
                n129 = Divide(x=w241, y=w247) -> (x/y=w246:dbl[])
                n130 = Multiply(x=w246, y=1000.0) -> (x*y=w243:dbl[])
                n131 = Bundle By Name(cluster=w244, "Image Dimension (um)"=w241, "Pixel Size (nm)"=w243) -> (w242:T16)
              }
              frame 4 {
                # "Pixel Size Change"
                n132 = Unbundle By Name(w259) -> ("Pixel Size (nm)"=w265:dbl[], "Image Format"=w263:u16, "Scan Mode"=w254:enum16{"XY", "XZ", "YZ", "XYZ"})
                n133 = for {
                  tunnel: w256 -> [w267] mode=indexing
                  tunnel: w265 -> [w266] mode=indexing
                  tunnel: [w266] -> w264
                  stop <- w267 stop-if-true
                }
                n134 = Build Array(w264, w264) -> (w258:dbl[])
                n135 = To Double Precision Float(number=w263) -> (double precision float=w262:dbl)
                n136 = Multiply(x=w258, y=w262) -> (x*y=w261:dbl[])
                n137 = Multiply(x=w261, y=0.001) -> (x*y=w255:dbl[])
                n138 = Bundle By Name(cluster=w259, "Pixel Size (nm)"=w258, "Image Dimension (um)"=w255) -> (w257:T16)
              }
            }
            n139 = Index Array(array=w208, index=0) -> (element=w232:dbl)
            n140 = Not Equal?(x=enum16{"XY", "XZ", "YZ", "XYZ"}."YZ" ("y"), y=w206) -> (x != y?=w217:bool)
            n141 = call "Res Mirror um to Volts.vi"("Image Size (um)"=w232) -> ("Voltage (V)"=w233:dbl)
            n142 = Select(t=15780.0, s=w217, f=200.0) -> (s? t:f=w220:dbl)
            n143 = In Range and Coerce(upper limit=5.0, x=w233, lower limit=0.0) -> (coerced(x)=w234:dbl)  [unwired: 1 out]
            n144 = Bundle By Name(cluster=w209, "Fast Axis Frequency (Hz)"=w220) -> (w219:T16)
            n145 = call "Volts to I16.vi"("Voltage (V)"=w234) -> ("I16"=w231:i16)  [unwired: 13 in, 1 out]
            n146 = call "Manual Controls Action Engine.vi"("Action"=enum16{"Read", "Write"}."Read") -> ("Manual Controls Out"=w225:T18)  [unwired: 14 in]
            n147 = Bundle By Name(cluster=w225, "Res Mirror Amp (I16)"=w231, "Res Mirror Mute"=w217) -> (w223:T18)
            n148 = call "Image Aquisition Param Ctrl_AE.vi"("Action"=enum16{"READ", "WRITE"}."WRITE", "Image Acquisition Parameters In"=w219) -> ()  [unwired: 9 in, 1 out]
            n149 = call "FPGA-7842R-Control V1.vi"("Action"=FPGA-7842R-Reference."Set Res Mirror", "Manual Controls"=w223, "Initialize"=TRUE) -> ()  [unwired: 11 in, 2 out]
            n150 = call "Manual Controls Action Engine.vi"("Action"=enum16{"Read", "Write"}."Write", "Manual Controls In"=w223) -> ()  [unwired: 13 in, 1 out]
          }
          frame "Detectors" {
            n151 = call "Detectors Crl_AE.vi"("Action"=enum16{"READ", "WRITE"}."WRITE", "Detectors Parameters In"="Detectors") -> ()  [unwired: 9 in, 1 out]
          }
          frame "Laser Controls" {
            w282 = FALSE ("element")
            n152 = Unbundle By Name("Laser Controls") -> ("STED"=w288:bool, "640 nm"=w285:bool, "590 nm"=w286:bool, "485 nm"=w287:bool, "STED Power (V)"=w279:dbl, "Manual Control"=w273:bool)
            n153 = local read "Live"() -> (w274:bool)
            n154 = call "LASERs_ Crl_AE.vi"("Action"=enum16{"READ", "WRITE"}."WRITE", "Detectors Parameters In"="Laser Controls") -> ()  [unwired: 9 in, 1 out]
            n155 = Or(x=w274, y=w273) -> (x .or. y?=w272:bool)
            n156 = In Range and Coerce(upper limit=10.0, x=w279, lower limit=0.0) -> (coerced(x)=w276:dbl)  [unwired: 1 out]
            n157 = Build Array(w288, w285, w286, w287, w282, w282, w282, w282) -> (w284:bool[])
            n158 = case shown="True" w272 {
              tunnel: "Laser Controls" -> [_ w294]
              frame False {
              }
              frame True {
                n159 = call "FPGA-7842R-Control V1.vi"("Action"=FPGA-7842R-Reference."Laser Control", "Laser Controls"=w294, "Initialize"=TRUE) -> ()  [unwired: 11 in, 2 out]
              }
            }
            n160 = Boolean Array To Number(Boolean array=w284) -> (number=w283:u32)
            n161 = To Unsigned Byte Integer(number=w283) -> (unsigned 8bit integer=w281:u8)
            n162 = call "U8_To_U32.vi"("U8 IN"=w281) -> ("U32 OUT"=w280:u32)  [unwired: 13 in, 1 out]
            n163 = call "Volts to I16.vi"("Voltage (V)"=w276) -> ("I16"=w275:i16)  [unwired: 13 in, 1 out]
            n164 = call "Scan Parameters Action Engine.vi"("Action"=enum16{"Read", "Write"}."Read") -> ("Scan Parameters OUT"=w291:T17)  [unwired: 14 in]
            n165 = Bundle By Name(cluster=w291, "Laser_States _U32"=w280, "775_AOM_Volt_I16"=w275) -> (w289:T17)
            n166 = call "Scan Parameters Action Engine.vi"("Action"=enum16{"Read", "Write"}."Write", "Scan Parameters IN"=w289) -> ()  [unwired: 13 in, 1 out]
          }
          frame "Shutters" {
            n167 = Unbundle By Name("Shutters") -> ("Upper Shutter"=w306:bool, "Lower Shutter"=w305:bool)
            n168 = Not(x=w306) -> (.not. x?=w297:bool)
            n169 = Not(x=w305) -> (.not. x?=w296:bool)
            n170 = call "Manual Controls Action Engine.vi"("Action"=enum16{"Read", "Write"}."Read") -> ("Manual Controls Out"=w301:T18)  [unwired: 14 in]
            n171 = Bundle By Name(cluster=w301, "Upper Shutter"=w297, "Lower Shutter"=w296) -> (w298:T18)
            n172 = call "Manual Controls Action Engine.vi"("Action"=enum16{"Read", "Write"}."Write", "Manual Controls In"=w298) -> ()  [unwired: 13 in, 1 out]
            n173 = call "FPGA-7842R-Control V1.vi"("Action"=FPGA-7842R-Reference."Shutter Control", "Manual Controls"=w298, "Initialize"=TRUE) -> ()  [unwired: 11 in, 2 out]
          }
        }
      }
      event Value Change {
        # "For P541 - Sample Z - Converting from Step in µm to I16 is as follows. We have (Step µw)*(10 V / 100 µm)*(32768 I16 / 10 V) = (Step µm)*(32768 I16 / 100 µm) = (Step µm)*(327.68 I16/µm)"
        n174 = event-data() -> ("CtlRef"=w321:refnum<vi>, "OldVal"=w319:variant, "NewVal"=w320:variant)  [unwired: 1 in]
        n175 = local write "Abort AllStage"(FALSE ("Abort AllStage")) -> ()
        n176 = property class="Clust"(reference=w321) -> ("Label.Text"=w318:string, "ClassName"=w307:string)  [unwired: 1 in, 2 out]
        n177 = case shown="\"Upper Objective Z - N664\"" w318 {
          tunnel: w320 -> [_ w344 w372 w399 w462 w489 w515]
          tunnel: w319 -> [_ w343 w371 w398 w463 w490 w516]
          tunnel: ["" "N664" "ASI" "P612" "P612" "P841" "M227"] -> w317
          tunnel: [dbl[] [0.0] w335 w364 w387 dbl[] [0.0] w478 w505] -> w316
          tunnel: [bool[] [FALSE] w333 w358 w388 bool[] [FALSE] bool[] [TRUE] w507] -> w315
          tunnel: [enum16{"MOVE", "MVR"}."MVR" ("MOVE/MVR") w332 w361 w390 enum16{"MOVE", "MVR"}."MVR" ("MOVE/MVR") w481 enum16{"MOVE", "MVR"}."MVR" ("MOVE/MVR")] -> w314
          tunnel: [0.0 ("Step Size (um)") 0.5 ("Step Size (um)") w363 0.0 ("Velocity") 0.0 ("Velocity") 10000.0 ("Velocity") 0.0 ("Velocity")] -> w310
          tunnel: [StageStates."MVR" ("Action") w330 w362 w391 StageStates."POSITION" ("Action") w482 StageStates."MVR" ("Action")] -> w308
          frame Default {
          }
          frame "Upper Objective Z - N664" {
            n178 = call "N664_Ctrl_Index.vi"("OldVal"=w343, "NewVal"=w344) -> ("Control Ref OUT"=w342:refnum<vi>, "N664 Out"=w340:T4)  [unwired: 12 in]
            n179 = property class="Ctl"(reference=w342) -> ("Label.Text"=w341:string)  [unwired: 1 in, 2 out]
            n180 = Unbundle By Name(w340) -> ("Step Size (um)"=w339:dbl, "Position (mm)"=w338:dbl)
            n181 = case shown="\"Down N664\"" w341 {
              tunnel: w339 -> [_ w350 w354 _]
              tunnel: [0.0 ("Step Size (um)") w350 w353 w357] -> w336
              tunnel: w338 -> [_ _ _ w357]
              tunnel: [enum16{"MOVE", "MVR"}."MVR" ("MOVE/MVR") enum16{"MOVE", "MVR"}."MVR" ("MOVE/MVR") enum16{"MOVE", "MVR"}."MVR" ("MOVE/MVR") enum16{"MOVE", "MVR"}."MOVE" ("MOVE/MVR")] -> w332
              tunnel: [StageStates."MVR" ("Action") StageStates."MVR" ("Action") StageStates."MVR" ("Action") StageStates."MOVE" ("Action")] -> w330
              frame Default {
              }
              frame "Up N664" {
              }
              frame "Down N664" {
                n182 = Negate(x=w354) -> (-x=w353:dbl)
              }
              frame "Position (mm)" {
              }
            }
            n183 = Build Array(w336) -> (w335:dbl[])
            n184 = Build Array(TRUE) -> (w333:bool[])
          }
          frame "Cavity Translation Z - ASI" {
            n185 = call "ASI_Ctrl_Index.vi"("NewVal"=w372, "OldVal"=w371) -> ("ASI out"=w368:T5, "Control Ref OUT"=w370:refnum<vi>)  [unwired: 8 in]
            n186 = property class="Ctl"(reference=w370) -> ("Label.Text"=w369:string)  [unwired: 1 in, 2 out]
            n187 = Unbundle By Name(w368) -> ("Step Size (um)"=w367:dbl, "Z (um)"=w366:dbl, "Velocity"=w363:dbl)
            n188 = case shown="\"Down ASI\"" w369 {
              tunnel: w367 -> [_ w378 w381 _]
              tunnel: w366 -> [_ _ _ w385]
              tunnel: [0.0 ("Z (um)") w378 w382 w385] -> w365
              tunnel: [StageStates."MVR" ("Action") StageStates."MVR" ("Action") StageStates."MVR" ("Action") StageStates."MOVE" ("Action")] -> w362
              tunnel: [enum16{"MOVE", "MVR"}."MVR" ("MOVE/MVR") enum16{"MOVE", "MVR"}."MVR" ("MOVE/MVR") enum16{"MOVE", "MVR"}."MVR" ("MOVE/MVR") enum16{"MOVE", "MVR"}."MOVE" ("MOVE/MVR")] -> w361
              frame Default {
              }
              frame "Up ASI" {
              }
              frame "Down ASI" {
                n189 = Negate(x=w381) -> (-x=w382:dbl)
              }
              frame "Z (um)" {
              }
            }
            n190 = Build Array(w365) -> (w364:dbl[])
            n191 = Build Array(TRUE) -> (w358:bool[])
          }
          frame "Bottom Objective XY - P612" {
            n192 = call "P612_Ctrl_Index.vi"("OldVal"=w398, "NewVal"=w399) -> ("Control out"=w397:refnum<vi>, "P612 out"=w395:T8)  [unwired: 12 in]
            n193 = property class="Ctl"(reference=w397) -> ("Label.Text"=w396:string)  [unwired: 1 in, 2 out]
            n194 = Unbundle By Name(w395) -> ("Step Size (um)"=w394:dbl, "X"=w393:dbl, "Y"=w392:dbl)
            n195 = case shown="\"Up Button\"" w396 {
              tunnel: w394 -> [_ _ w410 w417 w421 w428 _]
              tunnel: w393 -> [_ _ _ _ _ _ w435]
              tunnel: w392 -> [_ _ _ _ _ _ w434]
              tunnel: [StageStates."MVR" ("Action") StageStates."HOME" ("Action") StageStates."MVR" ("Action") StageStates."MVR" ("Action") StageStates."MVR" ("Action") StageStates."MVR" ("Action") StageStates."MOVE" ("Action")] -> w391
              tunnel: [enum16{"MOVE", "MVR"}."MVR" ("MOVE/MVR") enum16{"MOVE", "MVR"}."MVR" ("MOVE/MVR") enum16{"MOVE", "MVR"}."MVR" ("MOVE/MVR") enum16{"MOVE", "MVR"}."MVR" ("MOVE/MVR") enum16{"MOVE", "MVR"}."MVR" ("MOVE/MVR") enum16{"MOVE", "MVR"}."MVR" ("MOVE/MVR") enum16{"MOVE", "MVR"}."MOVE" ("MOVE/MVR")] -> w390
              tunnel: [bool[] [FALSE] bool[] [TRUE, TRUE] bool[] [TRUE, FALSE] bool[] [TRUE, FALSE] bool[] [FALSE, TRUE] bool[] [FALSE, TRUE] bool[] [TRUE, TRUE]] -> w388
              tunnel: [dbl[] [0.0] dbl[] [0.0, 0.0] w409 w416 w423 w430 w436] -> w387
              frame Default {
              }
              frame "Home Button" {
              }
              frame "Up Button" {
                n196 = Build Array(w410, 0.0 ("element")) -> (w409:dbl[])
              }
              frame "Down Button" {
                n197 = Negate(x=w417) -> (-x=w414:dbl)
                n198 = Build Array(w414, 0.0 ("element")) -> (w416:dbl[])
              }
              frame "Left Button" {
                n199 = Build Array(0.0 ("element"), w421) -> (w423:dbl[])
              }
              frame "Right Button" {
                n200 = Negate(x=w428) -> (-x=w427:dbl)
                n201 = Build Array(0.0 ("element"), w427) -> (w430:dbl[])
              }
              frame "X", "Y" {
                n202 = Build Array(w435, w434) -> (w436:dbl[])
              }
            }
          }
          frame "Sample Z - P541" {
            w455 = 327.68 ("y")
            n203 = call "P541_Ctrl_Index.vi"("OldVal"=w463, "NewVal"=w462) -> ("Control out"=w461:refnum<vi>, "P541 Out"=w460:T13)  [unwired: 12 in]
            n204 = property class="Ctl"(reference=w461) -> ("Label.Text"=w458:string)  [unwired: 1 in, 2 out]
            n205 = Unbundle By Name(w460) -> ("Z Position"=w456:dbl, "Step Size (um)"=w459:dbl)
            n206 = call "Manual Controls Action Engine.vi"("Action"=enum16{"Read", "Write"}."Read") -> ("Manual Controls Out"=w447:T18)  [unwired: 14 in]
            n207 = Unbundle By Name(w447) -> ("Z Axis Voltage (I16)"=w450:i16)
            n208 = Multiply(x=w455, y=w456) -> (x*y=w453:dbl)
            n209 = Multiply(x=w459, y=w455) -> (x*y=w457:dbl)
            n210 = Round To Nearest(number=w453) -> (nearest integer value=w442:dbl)
            n211 = Round To Nearest(number=w457) -> (nearest integer value=w441:dbl)
            n212 = To Word Integer(number=w442) -> (16bit integer=w452:i16)
            n213 = To Word Integer(number=w441) -> (16bit integer=w454:i16)
            n214 = case shown="\"Step Down\"" w458 {
              tunnel: w454 -> [_ w470 w474 _]
              tunnel: w452 -> [_ _ _ w476]
              tunnel: w450 -> [w469 w472 w475 _]
              tunnel: [w469 w471 w473 w476] -> w446
              frame Default {
              }
              frame "Step Down" {
                n215 = Subtract(x=w472, y=w470) -> (x-y=w471:i16)
              }
              frame "Step Up" {
                n216 = Add(x=w475, y=w474) -> (x+y=w473:i16)
              }
              frame "Z Position" {
              }
            }
            n217 = Bundle By Name(cluster=w447, "Z Axis Voltage (I16)"=w446) -> (w449:T18)
            n218 = call "Manual Controls Action Engine.vi"("Action"=enum16{"Read", "Write"}."Write", "Manual Controls In"=w449) -> ("Manual Controls Out"=w443:T18)  [unwired: 13 in]
            n219 = call "FPGA-7842R-Control V1.vi"("Action"=FPGA-7842R-Reference."Stage Control", "Manual Controls"=w443, "Initialize"=TRUE) -> ()  [unwired: 11 in, 2 out]
          }
          frame "Phase Comp Mirror - P841" {
            n220 = call "P841_Ctrl_Index.vi"("OldVal"=w490, "NewVal"=w489) -> ("Control out"=w487:refnum<vi>, "P841 Out"=w485:T6)  [unwired: 12 in]
            n221 = property class="Ctl"(reference=w487) -> ("Label.Text"=w486:string)  [unwired: 1 in, 2 out]
            n222 = Unbundle By Name(w485) -> ("Position (µm)"=w484:dbl, "Step Size (µm)"=w483:dbl)
            n223 = case shown="\"Down P841\"" w486 {
              tunnel: w484 -> [_ _ _ w503]
              tunnel: w483 -> [_ w496 w500 _]
              tunnel: [0.0 ("Position (µm)") w496 w499 w503] -> w479
              tunnel: [StageStates."MVR" ("Action") StageStates."MVR" ("Action") StageStates."MVR" ("Action") StageStates."MOVE" ("Action")] -> w482
              tunnel: [enum16{"MOVE", "MVR"}."MVR" ("MOVE/MVR") enum16{"MOVE", "MVR"}."MVR" ("MOVE/MVR") enum16{"MOVE", "MVR"}."MVR" ("MOVE/MVR") enum16{"MOVE", "MVR"}."MOVE" ("MOVE/MVR")] -> w481
              frame Default {
              }
              frame "Up P841" {
              }
              frame "Down P841" {
                n224 = Negate(x=w500) -> (-x=w499:dbl)
              }
              frame "Position (µm)" {
              }
            }
            n225 = Build Array(w479) -> (w478:dbl[])
          }
          frame "Sample Z Coarse - M227" {
            n226 = call "M227_Ctrl_Index.vi"("OldVal"=w516, "NewVal"=w515) -> ("Control Ref OUT"=w514:refnum<vi>, "M227 Out"=w512:T10)  [unwired: 12 in]
            n227 = property class="Ctl"(reference=w514) -> ("Label.Text"=w513:string)  [unwired: 1 in, 2 out]
            n228 = Unbundle By Name(w512) -> ("Step Size (mm)"=w511:dbl)
            n229 = case shown="\"Down M227\"" w513 {
              tunnel: w511 -> [_ w519 w522]
              tunnel: [bool[] [FALSE, FALSE, FALSE] bool[] [TRUE, TRUE, TRUE] bool[] [TRUE, TRUE, TRUE]] -> w507
              tunnel: [0.0 ("Step Size (mm)") w519 w521] -> w506
              frame Default {
              }
              frame "Up M227" {
              }
              frame "Down M227" {
                n230 = Negate(x=w522) -> (-x=w521:dbl)
              }
            }
            n231 = Build Array(w506) -> (w505:dbl[])
          }
        }
        n232 = case shown="\"Upper Objective Z - N664\"" w318 {
          tunnel: w307 -> [_ w524 _]
          frame Default {
          }
          frame "Upper Objective Z - N664" {
            n233 = case shown="\"Boolean\", Default" w524 {
              frame "Digital" {
                n234 = while {
                  shift-right: [w526] -> _
                  shift-left: TRUE ("Status Out") -> [w531]
                  stop <- w530 stop-if-true
                  n235 = call "Stage_position_ae.vi"("StageID"="N664", "Enum"=enum16{"WRITE", "READ"}."READ") -> ("Status Out"=w526:bool, "Position Out"=w536:dbl[])  [unwired: 8 in]
                  n236 = Greater?(x=w526, y=w531) -> (0:w530:bool)
                  n237 = Wait (ms)(milliseconds to wait=u32 1) -> ()  [unwired: 1 out]
                  n238 = Index Array(array=w536, index=0) -> (element=w535:dbl)
                  n239 = Select(t=u32 16777215, s=w526, f=u32 6618880) -> (s? t:f=w527:u32)
                  n240 = property on="Position (mm)" class="DigNum (strict)"("Value"=w535, "NumText.BG Color"=w527) -> ()  [unwired: 2 in, 2 out]
                }
              }
              frame "Boolean", Default {
              }
            }
          }
          frame "Cavity Translation Z - ASI" {
            n241 = while {
              shift-right: [w539] -> _
              shift-left: TRUE ("Status Out") -> [w544]
              stop <- w543 stop-if-true
              n242 = call "Stage_position_ae.vi"("StageID"="ASI", "Enum"=enum16{"WRITE", "READ"}."READ") -> ("Status Out"=w539:bool, "Position Out"=w549:dbl[])  [unwired: 8 in]
              n243 = Greater?(x=w539, y=w544) -> (0:w543:bool)
              n244 = Wait (ms)(milliseconds to wait=u32 1) -> ()  [unwired: 1 out]
              n245 = Index Array(array=w549, index=0) -> (element=w548:dbl)
              n246 = Select(t=u32 16777215, s=w539, f=u32 6618880) -> (s? t:f=w540:u32)
              n247 = property on="Z (um)" class="DigNum (strict)"("Value"=w548, "NumText.BG Color"=w540) -> ()  [unwired: 2 in, 2 out]
            }
          }
        }
        n248 = control-ref of="Abort AllStage"() -> (w309:refnum<vi>)
        n249 = call "AllStage_Limits_Array.vi"("Step(um)/Position(units)"=w316, "Axis"=w315, "Stage ID"=w317, "MOVE/MVR"=w314) -> ("Positions"=w312:dbl[], "Boolean Array"=w311:bool[], "Stage ID"=w313:string)  [unwired: 5 in]
        n250 = call "AE_AllStages_Action V2.vi"("Velocity"=w310, "Abort"=w309, "Positions"=w312, "Axis"=w311, "Stage ID"=w313, "Action"=w308) -> ()  [unwired: 3 in, 3 out]
      }
      event "SLM", "Timing", "DM": Value Change {
        n251 = event-data() -> ("CtlRef"=w554:refnum<vi>, "NewVal"=w551:bool)  [unwired: 1 in, 1 out]
        n252 = property class="Bool (strict)"(reference=w554) -> ("Label.Text"=w553:string)  [unwired: 1 in, 2 out]
        n253 = case shown="\"DM\"" w553 {
          tunnel: w551 -> [w555 w569 w583]
          frame "SLM", Default {
            n254 = case shown="False" w555 {
              frame False {
                n255 = To Variant(anything=TRUE) -> (Variant=w561:variant)
                n256 = call "SLM AE.vi"("Action"=enum16{"READ", "WRITE"}."READ") -> ("SLM Ref Out"=w562:refnum<vi>)  [unwired: 10 in]
                n257 = invoke class="VI" method="Ctrl Val.Set"(reference=w562, "Control Name"="Exit", "Value"=w561) -> (reference out=w558:refnum<vi>, error out=w557:errorcluster)  [unwired: 2 in, 3 out]
                n258 = invoke on="Hamamatsu LCOS" class="SubPnl" method="Remove VI"(error in=w557) -> (error out=w556:errorcluster)  [unwired: 2 in, 2 out]
                n259 = Close Reference(reference=w558, error in (no error)=w556) -> ()  [unwired: 1 out]
              }
              frame True {
                n260 = Open VI Reference(vi path=path "C:/Users/ED STED/Documents/Test Control Software/Host VIs/SLM/SLM Control.vi") -> (vi reference=w567:refnum<vi>)  [unwired: 5 in, 1 out]
                n261 = invoke class="VI" method="Run VI"(reference=w567, "Wait until done"=FALSE ("Wait Until Done")) -> (reference out=w564:refnum<vi>)  [unwired: 3 in, 4 out]
                n262 = invoke on="Hamamatsu LCOS" class="SubPanel" method="Insert VI"("VI Ref"=w564) -> ()  [unwired: 3 in, 4 out]
                n263 = call "SLM AE.vi"("Action"=enum16{"READ", "WRITE"}."WRITE", "SLM Ref In"=w564) -> ()  [unwired: 9 in, 1 out]
              }
            }
          }
          frame "DM" {
            n264 = case shown="True" w569 {
              frame False {
                n265 = call "DM_Ref_AE.vi"("Action"=enum16{"READ", "WRITE"}."READ") -> ("DM Ref Out"=w576:refnum<vi>)  [unwired: 10 in]
                n266 = To Variant(anything=TRUE) -> (Variant=w575:variant)
                n267 = invoke class="VI" method="Ctrl Val.Set"(reference=w576, "Control Name"="Exit", "Value"=w575) -> (reference out=w572:refnum<vi>, error out=w571:errorcluster)  [unwired: 2 in, 3 out]
                n268 = invoke on="Hamamatsu LCOS" class="SubPnl" method="Remove VI"(error in=w571) -> (error out=w570:errorcluster)  [unwired: 2 in, 2 out]
                n269 = Close Reference(reference=w572, error in (no error)=w570) -> ()  [unwired: 1 out]
              }
              frame True {
                n270 = Open VI Reference(vi path=path "C:/Users/ED STED/Documents/Test Control Software/Host VIs/DM/DM_Control_STED.vi") -> (vi reference=w581:refnum<vi>)  [unwired: 5 in, 1 out]
                n271 = invoke class="VI" method="Run VI"(reference=w581, "Wait until done"=FALSE ("Wait Until Done")) -> (reference out=w578:refnum<vi>)  [unwired: 3 in, 4 out]
                n272 = invoke on="BM Multi" class="SubPanel" method="Insert VI"("VI Ref"=w578) -> ()  [unwired: 3 in, 4 out]
                n273 = call "DM_Ref_AE.vi"("Action"=enum16{"READ", "WRITE"}."WRITE", "DM Ref In"=w578) -> ()  [unwired: 9 in, 1 out]
              }
            }
          }
          frame "Timing" {
            n274 = case shown="True" w583 {
              frame False {
                n275 = To Variant(anything=TRUE) -> (Variant=w588:variant)
                n276 = call "GateDelay AE.vi"("Action"=enum16{"READ", "WRITE"}."READ") -> ("Gate Delay Ref Out"=w589:refnum<vi>)  [unwired: 10 in]
                n277 = invoke class="VI" method="Ctrl Val.Set"(reference=w589, "Control Name"="Exit", "Value"=w588) -> (reference out=w584:refnum<vi>, error out=w585:errorcluster)  [unwired: 2 in, 3 out]
                n278 = invoke on="Timing" class="SubPnl" method="Remove VI"(error in=w585) -> (error out=w591:errorcluster)  [unwired: 2 in, 2 out]
                n279 = Close Reference(reference=w584, error in (no error)=w591) -> ()  [unwired: 1 out]
              }
              frame True {
                n280 = Open VI Reference(vi path=path "C:/Users/ED STED/Documents/Test Control Software/Host VIs/Time Delay/GateDelay_Control_V1.vi") -> (vi reference=w594:refnum<vi>)  [unwired: 5 in, 1 out]
                n281 = invoke class="VI" method="Run VI"(reference=w594, "Wait until done"=FALSE ("Wait Until Done")) -> (reference out=w593:refnum<vi>)  [unwired: 3 in, 4 out]
                n282 = invoke on="Timing" class="SubPanel" method="Insert VI"("VI Ref"=w593) -> ()  [unwired: 3 in, 4 out]
                n283 = call "GateDelay AE.vi"("Action"=enum16{"READ", "WRITE"}."WRITE", "Gate Delay Ref In"=w593) -> ()  [unwired: 9 in, 1 out]
              }
            }
          }
        }
      }
      event Value Change {
        n284 = event-data() -> ("CtlRef"=w602:refnum<vi>, "OldVal"=w600:variant, "NewVal"=w599:variant)  [unwired: 1 in]
        n285 = property class="Clust"(reference=w602) -> ("Label.Text"=w601:string)  [unwired: 1 in, 2 out]
        n286 = call "Graph Ref AE.vi"("Action"=enum16{"READ", "WRITE"}."READ") -> ("Graph Ref Out"=w597:refnum<vi>[])  [unwired: 10 in]
        n287 = case shown="\"Graph Tools\"" w601 {
          tunnel: w600 -> [_ w609 w668]
          tunnel: w599 -> [_ w610 w667]
          tunnel: w597 -> [_ w604 w656]
          frame Default {
          }
          frame "Display Controls" {
            n288 = call "Display_Controls_Ctrl_Index.vi"("OldVal"=w609, "NewVal"=w610) -> ("Control Ref OUT"=w608:refnum<vi>, "Display Controls Out"=w606:T1)  [unwired: 12 in]
            n289 = property class="Ctl"(reference=w608) -> ("Label.Text"=w607:string)  [unwired: 1 in, 2 out]
            n290 = Unbundle By Name(w606) -> ("Single Screen"=w605:bool)
            n291 = case shown="\"Add Display\"" w607 {
              tunnel: w605 -> [w618 _ _]
              tunnel: w604 -> [_ w643 w650]
              frame "Single Screen", Default {
                n292 = property class="App"() -> ("Disp.AllMonitors"=w617:T29)  [unwired: 2 in, 2 out]
                n293 = Index Array(array=w617, index #1=1 ("index"), index #2=0 ("index")) -> (element #1=w614:T30, element #2=w613:T30)
                n294 = control-ref of="This VI"() -> (w612:refnum<vi>)
                n295 = case shown="True" w618 {
                  tunnel: w614 -> [w622 _]
                  tunnel: w613 -> [w621 w633]
                  tunnel: w612 -> [w620 w631]
                  tunnel: T22 {"Left"=0, "Top"=0, "Right"=0, "Bottom"=0} ("Front Panel Window:Window Bounds") -> [w619 w632]
                  frame False {
                    w627 = i16 0
                    n296 = Unbundle By Name(w621) -> ("Bounds.Left"=w624:i16, "Bounds.Bottom"=w625:i16, "Bounds.Top"=w626:i16)
                    n297 = Unbundle By Name(w622) -> ("Bounds.Right"=w623:i16)
                    n298 = Subtract(x=w623, y=w624) -> (x-y=w628:i16)
                    n299 = Subtract(x=w625, y=w626) -> (x-y=w629:i16)
                    n300 = Bundle By Name(cluster=w619, "Left"=w627, "Top"=w627, "Right"=w628, "Bottom"=w629) -> (w630:T22)
                    n301 = property class="VI"(reference=w620, "Front Panel.WinBounds"=w630) -> ()  [unwired: 1 in, 2 out]
                  }
                  frame True {
                    w636 = i16 0
                    n302 = Unbundle By Name(w633) -> ("Bounds.Right"=w639:i16, "Bounds.Bottom"=w638:i16, "Bounds.Top"=w637:i16)
                    n303 = Subtract(x=w638, y=w637) -> (x-y=w635:i16)
                    n304 = Bundle By Name(cluster=w632, "Left"=w636, "Top"=w636, "Right"=w639, "Bottom"=w635) -> (w634:T22)
                    n305 = property class="VI"(reference=w631, "Front Panel.WinBounds"=w634) -> (reference out=w641:refnum<vi>)  [unwired: 1 in, 1 out]
                    n306 = property class="VI"(reference=w641, "FP.State"=T23."Maximized" ("Front Panel Window:State")) -> ()  [unwired: 1 in, 2 out]
                  }
                }
              }
              frame "Add Display" {
                w644 = u16 0 items=["Read", "Write"] ("Action")
                w648 = u16 1 items=["Read", "Write"] ("Action")
                n307 = property on="Add Display" class="Bool (strict)"("Value"=FALSE) -> ()  [unwired: 2 in, 2 out]
                n308 = call "Arange_Displays_V2.vi"("Action"=w644) -> ("Number of Channels OUT"=w645:i32)  [unwired: 14 in]
                n309 = Increment(x=w645) -> (x+1=w647:i32)
                n310 = call "Arange_Displays_V2.vi"("Display References"=w643, "Action"=w648, "Number of Channels"=w647, "Aspect Ratio (h/w)"=1.0) -> ()  [unwired: 11 in, 1 out]
              }
              frame "Remove Display" {
                w651 = u16 0 items=["Read", "Write"] ("Action")
                w655 = u16 1 items=["Read", "Write"] ("Action")
                n311 = call "Arange_Displays_V2.vi"("Action"=w651) -> ("Number of Channels OUT"=w652:i32)  [unwired: 14 in]
                n312 = Decrement(x=w652) -> (x-1=w654:i32)
                n313 = call "Arange_Displays_V2.vi"("Display References"=w650, "Action"=w655, "Number of Channels"=w654, "Aspect Ratio (h/w)"=1.0) -> ()  [unwired: 11 in, 1 out]
                n314 = property on="Remove Display" class="Bool (strict)"("Value"=FALSE) -> ()  [unwired: 2 in, 2 out]
              }
            }
          }
          frame "Graph Tools" {
            n315 = call "Graph_Controls_Ctrl_Index.vi"("OldVal"=w668, "NewVal"=w667) -> ("Control Ref OUT"=w666:refnum<vi>, "Graph Tools Out"=w665:T2)  [unwired: 12 in]
            n316 = property class="Ctl"(reference=w666) -> (reference out=w658:refnum<vi>, "Label.Text"=w657:string)  [unwired: 1 in, 1 out]
            n317 = Unbundle By Name(w665) -> ("Show Cursor"=w664:bool, "Auto Scale"=w663:bool, "Zoom In"=w662:bool, "Zoom Out"=w661:bool, "Pan Tool"=w660:bool, "Reset Zoom"=w659:bool)
            n318 = case shown="\"Pan Tool\", \"Reset Zoom\", \"Zoom In\", \"Zoom Out\"" w657 {
              selector: w657 -> [_ _ w704 _ _ _ _]
              tunnel: w664 -> [w670 _ _ _ _ _ _]
              tunnel: w663 -> [_ w690 _ _ _ _ _]
              tunnel: w656 -> [w669 w691 w703 w724 _ w756 w764]
              tunnel: w662 -> [_ _ w708 _ _ _ _]
              tunnel: w661 -> [_ _ w705 _ _ _ _]
              tunnel: w660 -> [_ _ w706 _ _ _ _]
              tunnel: w659 -> [_ _ w707 _ _ _ _]
              tunnel: w658 -> [_ _ _ _ _ _ _]
              tunnel: w657 -> [_ _ w695 _ _ _ _]
              frame "Show Cursor", Default {
                w673 = 2.0 ("y")
                n319 = Index Array(array=w669, index=0) -> (element=w681:refnum<vi>)
                n320 = property class="IntGraph (strict)"(reference=w681) -> ("Value"=w680:sgl[][])  [unwired: 1 in, 2 out]
                n321 = Array Size(array=w680) -> (size(s)=w679:i32[])
                n322 = To Double Precision Float(number=w679) -> (double precision float=w676:dbl[])
                n323 = Index Array(array=w676, index #1=0 ("index"), index #2=1 ("index")) -> (element #1=w675:dbl, element #2=w674:dbl)
                n324 = Divide(x=w675, y=w673) -> (x/y=w672:dbl)
                n325 = Divide(x=w674, y=w673) -> (x/y=w671:dbl)
                n326 = for {
                  tunnel: w669 -> [w686] mode=indexing
                  tunnel: w672 -> [w684]
                  tunnel: w671 -> [w685]
                  tunnel: w670 -> [w683]
                  n327 = property class="IntGraph (strict)"(reference=w686, "Cursor.Visible"=w683, "Cursor.Cursor X"=w684, "Cursor.Cursor Y"=w685) -> ()  [unwired: 1 in, 2 out]
                }
              }
              frame "Auto Scale" {
                n328 = Select(t=u8 2 ("Z Scale.Scale Fit"), s=w690, f=u8 0) -> (s? t:f=w687:u8)
                n329 = for {
                  tunnel: w691 -> [w693] mode=indexing
                  tunnel: w687 -> [w692]
                  n330 = property class="IntGraph (strict)"(reference=w693, "ZScale.ScaleFit"=w692) -> ()  [unwired: 1 in, 2 out]
                }
              }
              frame "Pan Tool", "Reset Zoom", "Zoom In", "Zoom Out" {
                n331 = Compound Arithmetic op=OR(w708, w705, w706, w707) -> (w700:bool)
                n332 = case shown="\"Zoom In\"" w704 {
                  tunnel: [0 ("Palette:Active Tool") 6 ("Palette:Active Tool") 7 ("Palette:Active Tool") 1 ("Palette:Active Tool") 5 ("Palette:Active Tool")] -> w702
                  frame Default {
                  }
                  frame "Zoom In" {
                  }
                  frame "Zoom Out" {
                  }
                  frame "Pan Tool" {
                  }
                  frame "Reset Zoom" {
                    n333 = property on="Reset Zoom" class="Bool (strict)"("Value"=FALSE) -> ()  [unwired: 2 in, 2 out]
                  }
                }
                n334 = control-ref of="Zoom In"() -> (w696:refnum<vi>)
                n335 = control-ref of="Zoom Out"() -> (w698:refnum<vi>)
                n336 = control-ref of="Pan Tool"() -> (w697:refnum<vi>)
                n337 = Select(t=w702, s=w700, f=0) -> (s? t:f=w694:i32)
                n338 = for {
                  tunnel: w703 -> [w715] mode=indexing
                  tunnel: w694 -> [w714]
                  n339 = property class="IntGraph (strict)"(reference=w715, "ActPaletteTool"=w714) -> ()  [unwired: 1 in, 2 out]
                }
                n340 = Build Array(w696, w698, w697) -> (w699:refnum<vi>[])
                n341 = for {
                  tunnel: w699 -> [w713] mode=indexing
                  tunnel: w695 -> [w711]
                  n342 = property class="Bool (strict)"(reference=w713) -> (reference out=w712:refnum<vi>, "Label.Text"=w710:string)  [unwired: 1 in, 1 out]
                  n343 = Equal?(x=w710, y=w711) -> (x = y?=w709:bool)
                  n344 = property class="Bool (strict)"(reference=w712, "Value"=w709) -> ()  [unwired: 1 in, 2 out]
                }
              }
              frame "Load File" {
                w735 = u16 1 items=["Get Image", "Load and Read File"] ("Action")
                n345 = event shown="[0] \"Channel 1\", \"Channel 2\", \"Channel 3\", \"Channel 4\", \"Channel 5\", \"Channel 6\": Mouse Down" {
                  selector: _ -> [_]
                  dyn-events: _ -> [_]
                  timeout: _ -> [_]
                  tunnel: [w738] -> w725
                  tunnel: [u16 1 ("icon")] -> w723
                  event "Channel 1", "Channel 2", "Channel 3", "Channel 4", "Channel 5", "Channel 6": Mouse Down {
                    n346 = event-data() -> ("CtlRef"=w746:refnum<vi>)  [unwired: 1 in]
                    n347 = property class="IntGraph (strict)"(reference=w746) -> ("Label.Text"=w745:string)  [unwired: 1 in, 2 out]
                    n348 = Reverse String(1:w745) -> (0:w740:string)
                    n349 = String Subset(string=w740, offset (0)=0, length (rest)=1 ("length (rest)")) -> (substring=w742:string)
                    n350 = Decimal String To Number(string=w742, default (0L)=0 ("default (0 I32)")) -> (number=w739:i32)  [unwired: 1 in, 1 out]
                    n351 = Decrement(x=w739) -> (x-1=w738:i32)
                  }
                }
                n352 = call-poly <vilib>:"Set Cursor.vi"("icon"=u16 27) -> ()  [unwired: 9 in, 2 out]
                n353 = property on="Load File" class="Bool (strict)"("Value"=FALSE) -> ()  [unwired: 2 in, 2 out]
                n354 = call "OpenDBL.vi"("Action"=w735) -> ("Image"=w734:sgl[], "Dimensions (Z, Y, X, t)"=w733:i32[])  [unwired: 12 in, 1 out]
                n355 = Index Array(array=w733, index #1=1 ("index"), index #2=2 ("index")) -> (element #1=w730:i32, element #2=w729:i32)
                n356 = Reverse 1D Array(array=w734) -> (reversed array=w728:sgl[])
                n357 = Reshape Array(w728, w730, w729) -> (w727:sgl[][])
                n358 = Index Array(array=w724, index=w725) -> (element=w736:refnum<vi>)
                n359 = property class="IntGraph (strict)"(reference=w736, "Value"=w727) -> ()  [unwired: 1 in, 2 out]
                n360 = call-poly <vilib>:"Set Cursor.vi"("icon"=w723) -> ()  [unwired: 9 in, 2 out]
              }
              frame "Fit Tool" {
                n361 = disable-structure shown="Disabled" {
                  frame Disabled {
                    n362 = vi-ref "QuickProfile_V3.vi"() -> (w748:refnum<vi>)
                    n363 = property class="VI Interface Type 0"(reference=w748) -> ("Path"=w751:path)  [unwired: 1 in, 2 out]
                    n364 = Unbundle By Name() -> ("Pixel Size (nm)"=w747:dbl[])  [unwired: 1 in]
                    n365 = Index Array(array=w747, index=0) -> (element=w754:dbl)
                    n366 = Open VI Reference(type specifier VI Refnum (for type only)=w748, vi path=w751, options=128) -> (vi reference=w749:refnum<vi>)  [unwired: 3 in, 1 out]
                    n367 = call-by-ref "Start Asynchronous Call"(reference=w749, "Pixel Size (nm)"=w754) -> (reference out=w752:refnum<vi>)  [unwired: 16 in, 1 out]
                    n368 = Close Reference(reference=w752) -> ()  [unwired: 1 in, 1 out]
                  }
                  frame Enabled {
                  }
                }
              }
              frame "Smooth Tool" {
                n369 = vi-ref "SmoothTool.vi"() -> (w759:refnum<vi>)
                n370 = property on="Smooth Tool" class="Bool (strict)"("Value"=FALSE) -> ()  [unwired: 2 in, 2 out]
                n371 = property class="VI Interface Type 1"(reference=w759) -> ("Path"=w761:path)  [unwired: 1 in, 2 out]
                n372 = control-ref of="This VI"() -> (w757:refnum<vi>)
                n373 = Open VI Reference(type specifier VI Refnum (for type only)=w759, vi path=w761, options=128) -> (vi reference=w760:refnum<vi>)  [unwired: 3 in, 1 out]
                n374 = call-by-ref "Start Asynchronous Call"(reference=w760, "Calling VI REF"=w757, "Display REFs In"=w756) -> (reference out=w758:refnum<vi>)  [unwired: 11 in, 1 out]
                n375 = Close Reference(reference=w758) -> ()  [unwired: 1 in, 1 out]
              }
              frame "Merge Tool" {
                n376 = vi-ref "MergeTool - Cambridge.vi"() -> (w767:refnum<vi>)
                n377 = property class="VI Interface Type 2"(reference=w767) -> ("Path"=w769:path)  [unwired: 1 in, 2 out]
                n378 = property on="Merge Tool" class="Bool (strict)"("Value"=FALSE) -> ()  [unwired: 2 in, 2 out]
                n379 = control-ref of="This VI"() -> (w765:refnum<vi>)
                n380 = Open VI Reference(type specifier VI Refnum (for type only)=w767, vi path=w769, options=128) -> (vi reference=w768:refnum<vi>)  [unwired: 3 in, 1 out]
                n381 = call-by-ref "Start Asynchronous Call"(reference=w768, "VI Reference"=w765, "Display References"=w764) -> (reference out=w766:refnum<vi>)  [unwired: 11 in, 1 out]
                n382 = Close Reference(reference=w766) -> ()  [unwired: 1 in, 1 out]
              }
            }
          }
        }
      }
      event "Test": Value Change {
        n383 = event-data() -> ()  [unwired: 1 in, 6 out]
        n384 = call "Graph Ref AE.vi"("Action"=enum16{"READ", "WRITE"}."READ") -> ("Graph Ref Out"=w771:refnum<vi>[])  [unwired: 10 in]
        n385 = for {
          tunnel: w771 -> [w774] mode=indexing
          n386 = property class="IntGraph (strict)"(reference=w774, "ActPaletteTool"=0 ("Palette:Active Tool")) -> ()  [unwired: 1 in, 2 out]
        }
      }
      event "Load Positions": Value Change {
        n387 = event-data() -> ()  [unwired: 1 in, 6 out]
        n388 = call "Load Stage Positions.vi"() -> ("appended array"=w787:bool[])  [unwired: 1 in]
        n389 = control-ref of="Abort AllStage"() -> (w785:refnum<vi>)
        n390 = Build Array("P841", "M686", "M686", "P612") -> (w786:string[])
        n391 = TDMS Open(10:T24."open (read-only)" ("operation (0:open)"), 11:path "C:/Users/ED STED/Documents/Test Control Software/Host VIs/Stages/Stage Positions/Stage Positions in Last Experiment.tdms" ("file path")) -> (3:w781:refnum<k34>)  [unwired: 5 in, 1 out]
        n392 = TDMS Read(0:w781, 5:"Stage Positions" ("group name in (Untitled)")) -> (4:w780:refnum<k34>, 10:w778:waveform(dbl)[])  [unwired: 6 in, 4 out]
        n393 = Index Array(array=w778, index=0) -> (element=w776:waveform(dbl))
        n394 = TDMS Close(11:w780) -> ()  [unwired: 1 in, 2 out]
        n395 = Unbundle By Name(w776) -> ("Y"=w775:dbl[])
        n396 = for {
          N -> [w793]
          tunnel: w787 -> [w796] mode=indexing
          tunnel: w786 -> [w795] mode=indexing
          tunnel: w785 -> [w794]
          tunnel: w775 -> [w792] mode=indexing
          n397 = case shown="True" w796 {
            tunnel: w795 -> [_ w799]
            tunnel: w794 -> [_ w800]
            tunnel: w793 -> [_ w798]
            tunnel: w792 -> [_ w797]
            frame False {
            }
            frame True {
              n398 = case shown="\"M686\"" w799 {
                tunnel: w800 -> [w804 w828 w856]
                tunnel: w799 -> [w805 w829 w857]
                tunnel: w798 -> [_ w825 w853]
                tunnel: w797 -> [w802 w824 w852]
                frame "P612", Default {
                  n399 = flat-sequence {
                    tunnel: w805 -> [w816]
                    tunnel: w804 -> [w817]
                    tunnel: [w817] -> w803
                    tunnel: w802 -> [w806]
                    tunnel: [w816] -> w801
                    tunnel: w803 -> [w822]
                    tunnel: w801 -> [w819]
                    frame #0 {
                      n400 = Divide(x=w806, y=10.0) -> (x/y=w809:dbl)
                      n401 = call "Volts to I16.vi"("Voltage (V)"=w809) -> ("I16"=w810:i16)  [unwired: 13 in, 1 out]
                      n402 = call "Manual Controls Action Engine.vi"("Action"=enum16{"Read", "Write"}."Read") -> ("Manual Controls Out"=w811:T18)  [unwired: 14 in]
                      n403 = Bundle By Name(cluster=w811, "Z Axis Voltage (I16)"=w810) -> (w814:T18)
                      n404 = call "Manual Controls Action Engine.vi"("Action"=enum16{"Read", "Write"}."Write", "Manual Controls In"=w814) -> ()  [unwired: 13 in, 1 out]
                      n405 = call "FPGA-7842R-Control V1.vi"("Action"=FPGA-7842R-Reference."Stage Control", "Manual Controls"=w814, "Initialize"=TRUE) -> ()  [unwired: 11 in, 2 out]
                    }
                    frame #1 {
                      n406 = call "AE_AllStages_Action V2.vi"("Abort"=w822, "Axis"=bool[] [TRUE, TRUE, TRUE], "Stage ID"=w819, "Action"=StageStates."POSITION") -> ("Position Out"=w821:dbl[])  [unwired: 5 in, 2 out]
                      n407 = Index Array(array=w821, index=2) -> ()  [unwired: 1 out]
                    }
                  }
                }
                frame "M686" {
                  n408 = flat-sequence {
                    tunnel: w829 -> [w841]
                    tunnel: w828 -> [w836]
                    tunnel: [w836] -> w827
                    tunnel: [w834] -> w826
                    tunnel: w825 -> [w833]
                    tunnel: w824 -> [w830]
                    tunnel: w827 -> [w850]
                    tunnel: w826 -> [w848]
                    frame #0 {
                      w834 = bool[] [TRUE, TRUE] ("Axis")
                      n409 = call "AE_AllStages_Action V2.vi"("Abort"=w836, "Axis"=w834, "Stage ID"=w841, "Action"=StageStates."POSITION") -> ("Position Out"=w840:dbl[])  [unwired: 5 in, 2 out]
                      n410 = Subtract(x=w833, y=1) -> (x-y=w831:i32)
                      n411 = Replace Array Subset(array=w840, new element=w830, index=w831) -> (w839:dbl[])
                      n412 = call "AE_AllStages_Action V2.vi"("Velocity"=1.0, "Abort"=w836, "Positions"=w839, "Axis"=w834, "Stage ID"="M686", "Action"=StageStates."MOVE") -> ()  [unwired: 3 in, 3 out]
                    }
                    frame #1 {
                      n413 = call "AE_AllStages_Action V2.vi"("Abort"=w850, "Axis"=w848, "Stage ID"="M686", "Action"=StageStates."POSITION") -> ("Position Out"=w847:dbl[])  [unwired: 5 in, 2 out]
                      n414 = Index Array(array=w847, index #1=0 ("index"), index #2=1 ("index")) -> (element #1=w845:dbl, element #2=w843:dbl)
                      n415 = property on="X" class="DigNum (strict)"("Value"=w845) -> ()  [unwired: 2 in, 2 out]
                      n416 = property on="Y" class="DigNum (strict)"("Value"=w843) -> ()  [unwired: 2 in, 2 out]
                    }
                  }
                }
                frame "P841" {
                  n417 = flat-sequence {
                    tunnel: w857 -> [_]
                    tunnel: w856 -> [w862]
                    tunnel: [w862] -> w855
                    tunnel: [w860] -> w854
                    tunnel: w853 -> [_]
                    tunnel: w852 -> [w858]
                    tunnel: w855 -> [w870]
                    tunnel: w854 -> [w868]
                    frame #0 {
                      w860 = bool[] [TRUE] ("Axis")
                      n418 = Build Array(w858) -> (w859:dbl[])
                      n419 = call "AE_AllStages_Action V2.vi"("Velocity"=1.0, "Abort"=w862, "Positions"=w859, "Axis"=w860, "Stage ID"="P841", "Action"=StageStates."MOVE") -> ()  [unwired: 3 in, 3 out]
                    }
                    frame #1 {
                      n420 = call "AE_AllStages_Action V2.vi"("Abort"=w870, "Axis"=w868, "Stage ID"="P841", "Action"=StageStates."POSITION") -> ("Position Out"=w867:dbl[])  [unwired: 5 in, 2 out]
                      n421 = Index Array(array=w867, index #1=0 ("index")) -> (element #1=w865:dbl)  [unwired: 1 in, 1 out]
                      n422 = property on="Position (µm)" class="DigNum (strict)"("Value"=w865) -> ()  [unwired: 2 in, 2 out]
                    }
                  }
                }
              }
            }
          }
        }
      }
      event "Exit": Value Change {
        n423 = event-data() -> ("CtlRef"=w883:refnum<vi>, "NewVal"=w885:bool)  [unwired: 1 in, 1 out]
        n424 = disable-structure shown="Disabled" {
          frame Disabled {
            n425 = Two Button Dialog(message="Record the positions of piezo stages?", 1:"No" ("F button name (\"Cancel\")"), 2:"Yes" ("T button name (\"OK\")")) -> (T button?=w886:bool)
            n426 = case shown="True" w886 {
              frame False {
              }
              frame True {
                n427 = Build Array("P612" ("Stage ID"), "M686" ("Stage ID"), "P841" ("Stage ID")) -> (w894:string[])
                n428 = for {
                  tunnel: w894 -> [w901] mode=indexing
                  tunnel: [w900] -> w890 mode=concatenating
                  n429 = call "Stage_position_ae.vi"("StageID"=w901, "Enum"=enum16{"WRITE", "READ"}."READ") -> ("Position Out"=w900:dbl[])  [unwired: 8 in, 1 out]
                }
                n430 = TDMS Open(10:T24."create or replace" ("operation (0:open)"), 11:path "C:/Users/ED STED/Documents/Test Control Software/Host VIs/Stages/Stage Positions/Stage Positions in Last Experiment.tdms" ("file path")) -> (3:w896:refnum<k34>)  [unwired: 5 in, 1 out]
                n431 = TDMS Write(0:w896, 5:"Stage Positions" ("group name in (Untitled)"), 9:w890) -> (4:w897:refnum<k34>)  [unwired: 3 in, 3 out]
                n432 = TDMS Close(11:w897) -> ()  [unwired: 1 in, 2 out]
              }
            }
          }
          frame Enabled {
          }
        }
        n433 = Release Notifier(notifier=w878, force destroy? (F)=TRUE) -> ()  [unwired: 1 in, 3 out]
        n434 = property class="Bool"(reference=w883) -> ("Label.Text"=w882:string)  [unwired: 1 in, 2 out]
        n435 = call "SLM AE.vi"("Action"=enum16{"READ", "WRITE"}."READ") -> ("SLM Ref Out"=w876:refnum<vi>)  [unwired: 10 in]
        n436 = call "DM_Ref_AE.vi"("Action"=enum16{"READ", "WRITE"}."READ") -> ("DM Ref Out"=w874:refnum<vi>)  [unwired: 10 in]
        n437 = call "GateDelay AE.vi"("Action"=enum16{"READ", "WRITE"}."READ") -> ("Gate Delay Ref Out"=w875:refnum<vi>)  [unwired: 10 in]
        n438 = Enqueue Element(queue=w884, element=w882) -> ()  [unwired: 2 in, 3 out]
        n439 = Build Array(w876, w874, w875) -> (w873:refnum<vi>[])
        n440 = for {
          tunnel: w873 -> [w907] mode=indexing
          n441 = Not A Number/Path/Refnum?(number/path/refnum=w907) -> (NaN/Path/Refnum?=w906:bool)
          n442 = case shown="False" w906 {
            tunnel: w907 -> [w908 _]
            frame False {
              n443 = To Variant(anything=TRUE) -> (Variant=w909:variant)
              n444 = invoke class="VI" method="Ctrl Val.Set"(reference=w908, "Control Name"="Exit", "Value"=w909) -> (reference out=w912:refnum<vi>)  [unwired: 2 in, 4 out]
              n445 = Close Reference(reference=w912) -> ()  [unwired: 1 in, 1 out]
            }
            frame True {
            }
          }
        }
        n446 = property on="Stages" class="Clust (strict)"() -> ("Controls[]"=w872:refnum<vi>[])  [unwired: 2 in, 2 out]
        n447 = for {
          tunnel: w872 -> [w905] mode=indexing
          n448 = property class="Ctl"(reference=w905) -> ("Label.Text"=w904:string)  [unwired: 1 in, 2 out]
          n449 = call "All_Stages_Aloha.vi"("Aloha"=FALSE, "Stage ID"=w904) -> ()  [unwired: 9 in, 1 out]
        }
      }
    }
  }
  n450 = disable-structure shown="Disabled" {
    frame Disabled {
    }
    frame Enabled {
    }
  }
  n451 = call "Manual Controls Action Engine.vi"("Action"=enum16{"Read", "Write"}."Write", "Manual Controls In"=w27) -> ("Manual Controls Out"=w29:T18)  [unwired: 13 in]
  n452 = call "FPGA-7842R-Control V1.vi"("Action"=FPGA-7842R-Reference."Initialize", "Manual Controls"=w29, "Initialize"=FALSE) -> ("Initalized"=w9:bool)  [unwired: 11 in, 1 out]
  n453 = while {
    shift-right: [w922] -> _
    shift-left: "Idle" -> [w923]
    tunnel: w16 -> [w919]
    shift-right: [w917] -> _
    shift-left: w9 -> [w918]
    stop <- w921 stop-if-true
    n454 = call "Image Aquisition Param Ctrl_AE.vi"("Action"=enum16{"READ", "WRITE"}."READ") -> ("Image Acquisition Parameters Out"=w916:T16)  [unwired: 10 in]
    n455 = call "Detectors Crl_AE.vi"("Action"=enum16{"READ", "WRITE"}."READ") -> ("Detectors Parameters Out"=w914:T14)  [unwired: 10 in]
    n456 = case shown="\"Display\"" w923 {
      selector: w923 -> [_ _ _ w955 _ _ _ _ _ _]
      tunnel: ["Exit" w932 "Idle" ("name (unnamed)") "Arange Displays" ("name (unnamed)") "Start FPGA Acquisition" ("name (unnamed)") "Display" ("name (unnamed)") "Close Images" ("name (unnamed)") "Idle" "Stop Waveforms" ("name (unnamed)") "Start Waveforms" ("name (unnamed)")] -> w922
      tunnel: [TRUE w934 w941 w963 w979 w1000 w1041 w1074 w1079 w1085] -> w921
      tunnel: FALSE -> [_ w934 w941 w963 w979 w1000 w1041 w1074 w1079 w1085]
      tunnel: w919 -> [_ w933 _ _ _ _ _ _ _ _]
      tunnel: w918 -> [w928 w931 w942 w961 w976 w998 w1039 w1072 w1080 w1086]
      tunnel: [w927 w931 w942 w961 w976 w994 w1039 w1071 w1080 w1086] -> w917
      tunnel: w916 -> [_ _ _ w954 _ w993 _ _ _ w1083]
      tunnel: w914 -> [_ _ _ w953 _ _ _ _ _ w1081]
      frame "Exit" {
        n457 = call "Graph Ref AE.vi"("Action"=enum16{"READ", "WRITE"}."READ") -> ("Graph Ref Out"=w925:refnum<vi>[])  [unwired: 10 in]
        n458 = call "FPGA-7842R-Control V1.vi"("Action"=FPGA-7842R-Reference."Close FPGA", "Initialize"=w928) -> ("Initalized"=w927:bool)  [unwired: 12 in, 1 out]
        n459 = Close Reference(reference=w925) -> ()  [unwired: 1 in, 1 out]
      }
      frame "Idle", Default {
        n460 = Dequeue Element(queue=w933, timeout in ms (-1)=-1) -> (element=w932:string)  [unwired: 1 in, 3 out]
      }
      frame "Close Images" {
        w937 = u16 0 items=["Read", "Write"] ("Mode")
        w938 = u16 0 items=["Write", "Read"] ("Mode")
        n461 = call "File Action V1.vi"("Mode"=w937) -> ("Files Open"=w936:bool)  [unwired: 12 in, 2 out]
        n462 = call "Image_Actions_V1.vi"("Mode"=w938, "Action"="Trash Images") -> ()  [unwired: 12 in, 2 out]
        n463 = case shown="True" w936 {
          frame False {
          }
          frame True {
            w944 = u16 1 items=["Read", "Write"] ("Mode")
            n464 = call "File Action V1.vi"("Action"="Close Files", "Mode"=w944) -> ()  [unwired: 11 in, 3 out]
          }
        }
      }
      frame "Capture", "Live" {
        w959 = u16 0 items=["Write", "Read"] ("Mode")
        n465 = Cluster To Array(cluster=w953) -> (array=w951:bool[])
        n466 = Index Array(array=w951, index=4) -> (element=w948:bool)
        n467 = Boolean To (0,1)(Boolean=w951) -> (0, 1=w952:i16[])
        n468 = Add Array Elements(numeric array=w952) -> (sum=w949:i16)
        n469 = To Long Integer(number=w949) -> (32bit integer=w946:i32)
        n470 = Unbundle By Name(w954) -> ("Image Format"=w956:u16)
        n471 = Select(t=1, s=w948, f=w946) -> (s? t:f=w945:i32)
        n472 = case shown="Default" w955 {
          tunnel: w954 -> [_ w965]
          tunnel: w945 -> [_ w964]
          frame Default {
          }
          frame "Capture" {
            w968 = u16 1 items=["Read", "Write"] ("Mode")
            n473 = call "File Action V1.vi"("Action"="Open Files", "Mode"=w968, "Image Acquisition Parameters"=w965, "File Path IN"="Save File Path", "Number of Channels"=w964) -> ("File Path OUT"=w966:path)  [unwired: 8 in, 2 out]
            n474 = local write "Save File Path"(w966) -> ()
          }
        }
        n475 = To Long Integer(number=w956) -> (32bit integer=w958:i32)
        n476 = Bundle(w958, w958) -> (w957:cluster{i32, i32})  [unwired: 1 in]
        n477 = call "Image_Actions_V1.vi"("Image Size (Pixels)"=w957, "Mode"=w959, "Number of Channels"=w945, "Action"="Create Images") -> ()  [unwired: 10 in, 2 out]
      }
      frame "Arange Displays" {
        w974 = u16 1 items=["Write", "Read"] ("Mode")
        w977 = u16 1 items=["Read", "Write"] ("Action")
        n478 = call "Graph Ref AE.vi"("Action"=enum16{"READ", "WRITE"}."READ") -> ("Graph Ref Out"=w970:refnum<vi>[])  [unwired: 10 in]
        n479 = call "Image_Actions_V1.vi"("Mode"=w974) -> ("Image REFs OUT"=w975:T32[])  [unwired: 13 in, 1 out]
        n480 = Array Size(array=w975) -> (size(s)=w973:i32)
        n481 = call "Arange_Displays_V2.vi"("Display References"=w970, "Action"=w977, "Number of Channels"=w973, "Aspect Ratio (h/w)"=1.0) -> ("Number of Channels OUT"=w971:i32)  [unwired: 11 in]
        n482 = for {
          N: w971 -> [_]
          tunnel: w970 -> [w981] mode=indexing
          tunnel: [w984] -> _ mode=indexing
          i -> [w982]
          n483 = property class="IntGraph (strict)"(reference=w981) -> ("Label.Text"=w986:string)  [unwired: 1 in, 2 out]
          n484 = Equal To 0?(x=w982) -> (x = 0?=w983:bool)
          n485 = case shown="True" w983 {
            tunnel: w981 -> [_ w987]
            frame False {
            }
            frame True {
              n486 = property class="IntGraph (strict)"(reference=w987, "ZScale.Visible"=TRUE ("Z Scale.Visible"), "ZScale.Position"=T31 {"Left"=2308, "Top"=-340} ("Z Scale.Position")) -> ()  [unwired: 1 in, 2 out]
            }
          }
          n487 = To Unsigned Word Integer(number=w982) -> (unsigned 16bit integer=w985:u16)
          n488 = Bundle("Label.Text"=w986, w985) -> (w984:cluster{"Label.Text":string, u16})  [unwired: 1 in]
        }
      }
      frame "Start Waveforms" {
        n489 = call "Initialize Waveforms V4.vi"("Image Acquisition Parameters"=w993) -> ("Waveform Data to FPGA"=w999:T33)  [unwired: 14 in]
        n490 = Unbundle By Name(w993) -> ("Scan Type"=w992:enum16{"Sample Scanning", "Beam Scanning"})
        n491 = call "FPGA-7842R-Control V1.vi"("Waveform Data"=w999, "Action"=FPGA-7842R-Reference."Start Waveforms", "Image Acquisition Parameters"=w993, "Initialize"=w998) -> ("Initalized"=w995:bool)  [unwired: 10 in, 1 out]
        n492 = Equal?(x=w992, y=enum16{"Sample Scanning", "Beam Scanning"}."Sample Scanning" ("Scan Type")) -> (x = y?=w990:bool)
        n493 = case shown="False" w990 {
          tunnel: w995 -> [w1001 w1006]
          tunnel: [w1001 w1005] -> w994
          frame False {
          }
          frame True {
            n494 = call "Scan Parameters Action Engine.vi"("Action"=enum16{"Read", "Write"}."Read") -> ("Scan Parameters OUT"=w1003:T17)  [unwired: 14 in]
            n495 = Unbundle By Name(w1003) -> ("Unused_Axis_I16"=w1002:i16)
            n496 = call "FPGA-7842R-Control V1.vi"("Action"=FPGA-7842R-Reference."Unused Axis I16", "Initialize"=w1006, "Unused Axis Offset (I16)"=w1002) -> ("Initalized"=w1005:bool)  [unwired: 11 in, 1 out]
          }
        }
      }
      frame "Display" {
        w1034 = u16 1 items=["Write", "Read"] ("Mode")
        n497 = call "Image_Actions_V1.vi"("Mode"=w1034) -> ("Image REFs OUT"=w1036:T32[])  [unwired: 13 in, 1 out]
        n498 = Array Size(array=w1036) -> (size(s)=w1032:i32)
        n499 = Decrement(x=w1032) -> (x-1=w1031:i32)
        n500 = for {
          N: 6 -> [_]
          tunnel: w1031 -> [w1069]
          tunnel: [w1067] -> w1035 mode=indexing
          i -> [w1068]
          n501 = Greater Or Equal?(x=w1069, y=w1068) -> (x >= y?=w1067:bool)
        }
        n502 = Obtain Notifier(name (unnamed)="Running", notification data type=FALSE) -> (notifier out=w1008:refnum<notifier>)  [unwired: 2 in, 2 out]
        n503 = Index Array(array=w1035, index #1=1 ("index"), index #2=2 ("index"), index #3=3 ("index"), index #4=4 ("index"), index #5=5 ("index")) -> (element #1=w1020:bool, element #2=w1019:bool, element #3=w1018:bool, element #4=w1017:bool, element #5=w1016:bool)
        n504 = Index Array(array=w1036, index #1=0 ("index"), index #2=1 ("index"), index #3=2 ("index"), index #4=3 ("index"), index #5=4 ("index"), index #6=5 ("index")) -> (element #1=w1015:T32, element #2=w1014:T32, element #3=w1013:T32, element #4=w1012:T32, element #5=w1011:T32, element #6=w1010:T32)
        n505 = while {
          tunnel: w1020 -> [w1056]
          tunnel: w1019 -> [w1055]
          tunnel: w1018 -> [w1051]
          tunnel: w1017 -> [w1048]
          tunnel: w1016 -> [w1047]
          tunnel: w1015 -> [w1054]
          tunnel: w1014 -> [w1053]
          tunnel: w1013 -> [w1052]
          tunnel: w1012 -> [w1050]
          tunnel: w1011 -> [w1046]
          tunnel: w1010 -> [w1049]
          tunnel: w1008 -> [w1042]
          stop <- w1043 stop-if-true
          n506 = Get Notifier Status(notifier=w1042) -> (current notification=w1043:bool)  [unwired: 1 in, 4 out]
          n507 = case shown="False" w1056 {
            tunnel: w1053 -> [_ w1066]
            frame False {
            }
            frame True {
              n508 = call "IMAQ ImageToArray"("Image"=w1066) -> ("Image Pixels (Float)"=→"Channel 2":sgl[][])  [unwired: 3 in, 4 out]
            }
          }
          n509 = case shown="True" w1055 {
            tunnel: w1052 -> [_ w1064]
            frame False {
            }
            frame True {
              n510 = call "IMAQ ImageToArray"("Image"=w1064) -> ("Image Pixels (Float)"=→"Channel 3":sgl[][])  [unwired: 3 in, 4 out]
            }
          }
          n511 = call "IMAQ ImageToArray"("Image"=w1054) -> ("Image Pixels (Float)"=→"Channel 1":sgl[][])  [unwired: 3 in, 4 out]
          n512 = case shown="False" w1051 {
            tunnel: w1050 -> [_ w1062]
            frame False {
            }
            frame True {
              n513 = call "IMAQ ImageToArray"("Image"=w1062) -> ("Image Pixels (Float)"=→"Channel 4":sgl[][])  [unwired: 3 in, 4 out]
            }
          }
          n514 = case shown="False" w1048 {
            tunnel: w1046 -> [_ w1060]
            frame False {
            }
            frame True {
              n515 = call "IMAQ ImageToArray"("Image"=w1060) -> ("Image Pixels (Float)"=→"Channel 5":sgl[][])  [unwired: 3 in, 4 out]
            }
          }
          n516 = case shown="False" w1047 {
            tunnel: w1049 -> [_ w1058]
            frame False {
            }
            frame True {
              n517 = call "IMAQ ImageToArray"("Image"=w1058) -> ("Image Pixels (Float)"=→"Channel 6":sgl[][])  [unwired: 3 in, 4 out]
            }
          }
          n518 = Wait (ms)(milliseconds to wait=u32 100) -> ()  [unwired: 1 out]
        }
      }
      frame "Stop Waveforms" {
        n519 = call "FPGA-7842R-Control V1.vi"("Action"=FPGA-7842R-Reference."Stop Waveforms", "Initialize"=w1072) -> ("Initalized"=w1071:bool)  [unwired: 12 in, 1 out]
      }
      frame "Stop Acquisition" {
        n520 = call "FPGA-7842R-Control V1.vi"("Action"=FPGA-7842R-Reference."Laser Control", "Laser Controls"=T15 {"STED Power (V)"=0.0, "STED"=FALSE, "640 nm"=FALSE, "590 nm"=FALSE, "485 nm"=FALSE, "Manual Control"=FALSE} ("Laser Controls 2"), "Initialize"=TRUE) -> ()  [unwired: 11 in, 2 out]
      }
      frame "Start FPGA Acquisition" {
        n521 = Unbundle By Name(w1083) -> ("Scan Mode"=w1082:enum16{"XY", "XZ", "YZ", "XYZ"})
        n522 = case shown="\"XZ\", Default" w1082 {
          tunnel: w1083 -> [_ w1093]
          tunnel: w1081 -> [_ w1094]
          frame "YZ" {
            n523 = vi-ref "FPGA Sample Scanning V1.vi"() -> (w1089:refnum<vi>)
            n524 = property class="VI Interface Type 3"(reference=w1089) -> ("Path"=w1087:path)  [unwired: 1 in, 2 out]
            n525 = Open VI Reference(type specifier VI Refnum (for type only)=w1089, vi path=w1087, options=128) -> (vi reference=w1090:refnum<vi>)  [unwired: 3 in, 1 out]
            n526 = call-by-ref "Start Asynchronous Call"(reference=w1090) -> (reference out=w1091:refnum<vi>)  [unwired: 4 in, 1 out]
            n527 = Close Reference(reference=w1091) -> ()  [unwired: 1 in, 1 out]
          }
          frame "XZ", Default {
            n528 = vi-ref "FPGA Beam Scanning V1.vi"() -> (w1092:refnum<vi>)
            n529 = property class="VI Interface Type 4"(reference=w1092) -> ("Path"=w1096:path)  [unwired: 1 in, 2 out]
            n530 = Open VI Reference(type specifier VI Refnum (for type only)=w1092, vi path=w1096, options=128) -> (vi reference=w1095:refnum<vi>)  [unwired: 3 in, 1 out]
            n531 = call-by-ref "Start Asynchronous Call"(reference=w1095, "Detectors"=w1094, "Image Acquisition Parameters"=w1093) -> (reference out=w1098:refnum<vi>)  [unwired: 2 in, 1 out]
            n532 = Close Reference(reference=w1098) -> ()  [unwired: 1 in, 1 out]
          }
        }
      }
    }
  }
